vi "DB UI - Admin User.vi"() -> ()   [LabVIEW 2013]
uses:
  Controls/Combo Box.ctl
  <vilib>/Utility/miscctls.llb/LVRowAndColumnUnsignedTypeDef.ctl
  <vilib>/Utility/miscctls.llb/LVRowAndColumnTypeDef.ctl
  <vilib>/Utility/miscctls.llb/LVPointTypeDef.ctl
  Controls/DB - Admin User Query ColNames.ctl
  Controls/Logon - Enum.ctl
  Controls/Global SRTRS.vi
  Controls/Global CMS.vi
  Controls/Global AMS.vi
  <vilib>/addons/database/Connection.llb/DB Tools Open Connec (String).vi
  <vilib>/addons/database/Connection.llb/Conn Execute.vi
  <vilib>/addons/database/Recordset.llb/Rec Destroy - Connection.vi
  <vilib>/addons/database/Recordset.llb/Rec Fetch Recordset Data (R).vi
  <vilib>/addons/database/_DB Variant To Data/Database Variant To Data.xnode
  <vilib>/addons/database/NI_Database_API.lvlib
panel:
  in  "Application":string
  in  "List [CaptionOnly]":string caption="List"
  in  "Tab Control":enum32{"Debug"}(tab)
  in  "DB.Config.UserGroup":string="SRTRS.Config.UserGroup"
  in  "DB.Config.UserGroupRelation":string="SRTRS.Config.UserGroupRelation"
  out "Password Matched":bool
  out "Password Count Valid":bool
  out "Email Valid":bool
  out "MHandler":errorcluster
  out "Connection Information":T1={"Connection "="SQL Server 32bit HPEnvy", "Username"="admin", "Password"="admin123"}
  in  "Stop Button":bool
  out "Statemachine":errorcluster
  in  "# of Columns":i32=9
  out "Primary Keys":string[](array[string])=["OrderNo"]
  out "Foreign Keys":string[](array[string])=["OrderNo"]
  in  "Next Button":bool
  in  "Previous Button":bool
  out "1st Primary KEY":string
  in  "Last Button":bool
  in  "First Button":bool
  out "datetime string":string
  out "Changed":bool
  out "SQL Query":string
  in  "Include Inactive":bool=TRUE
  out "Extra Event From \"Select Foreign Key\"":bool
  out "IDENTITY COLUMN":string
  out "Close":errorcluster
  out "New Record in UI not in DB":bool
  out "Property Node":errorcluster
  out "DB":errorcluster
  in  "DB.Admin.Users":string="SRTRS.Admin.Users"
  out "Col INFO":string[][](array[string])
  in  "[PlantId]":string="4070"
  in  "DB.Config.TabUserAccess":string="SRTRS.Config.TabUserAccess" caption="DB.Schema.Table\nDB.Config.TabUserAccess"
  in  "DB.Config.UserStationAccess":string="SRTRS.Config.UserStationAccess"
  out "Col Hdrs[] DB Data Type":string[](array[string])
  in  "# of Rows":u32=11
  out "Col Hdrs[] DB Precision":string[](array[string])
  out "All Mandatory Fields Filled":bool
  in  "------------------------------------        User Details Header EVENTS     ------------------------------------":string caption="------------------------------------        Setup Tab     ------------------------------------"
  in  "------------------------------------------        Unused EVENTS     ----------------------------------------":string caption="------------------------------------        Setup Tab     ------------------------------------"
  out "Logon":errorcluster
  out "MCListBox":u32
  out "NewVal":i32
  out "User Details 2":u32
  out "Controls (Caption) that are blank (Unicode)":string[](array[string])
  in  "Save Enabled depends on \nFilled Mandatory Fields":bool
  in  "CellBG New Cells":u32(colorbox)=16777225
  in  "CellBG Unused Cells":u32(colorbox)=16777238
  in  "CellBG ColHdrs":u32(colorbox)=11776947
  in  "Ascending":bool
  out "transposed array":string[][](array[string])
  in  "DB.Config.Domain":string="SRTRS.Config.Domain"
  in  "DB.Config.Plant":string="SRTRS.Config.Plant"
  in  "Search User ID":T2
  in  "Save":bool caption="Setup Save"
  in  "New":bool caption="Setup Save"
  in  "User Details":T3 caption="Record"
  in  "Current Record":i32 caption="No."
  out "Record Count":i32
  in  "Multicolumn Listbox":i32(listbox)=3
  # "Cannot be placed in Tab, becasue calling VI only looking for non-Tabs."
  # "/"
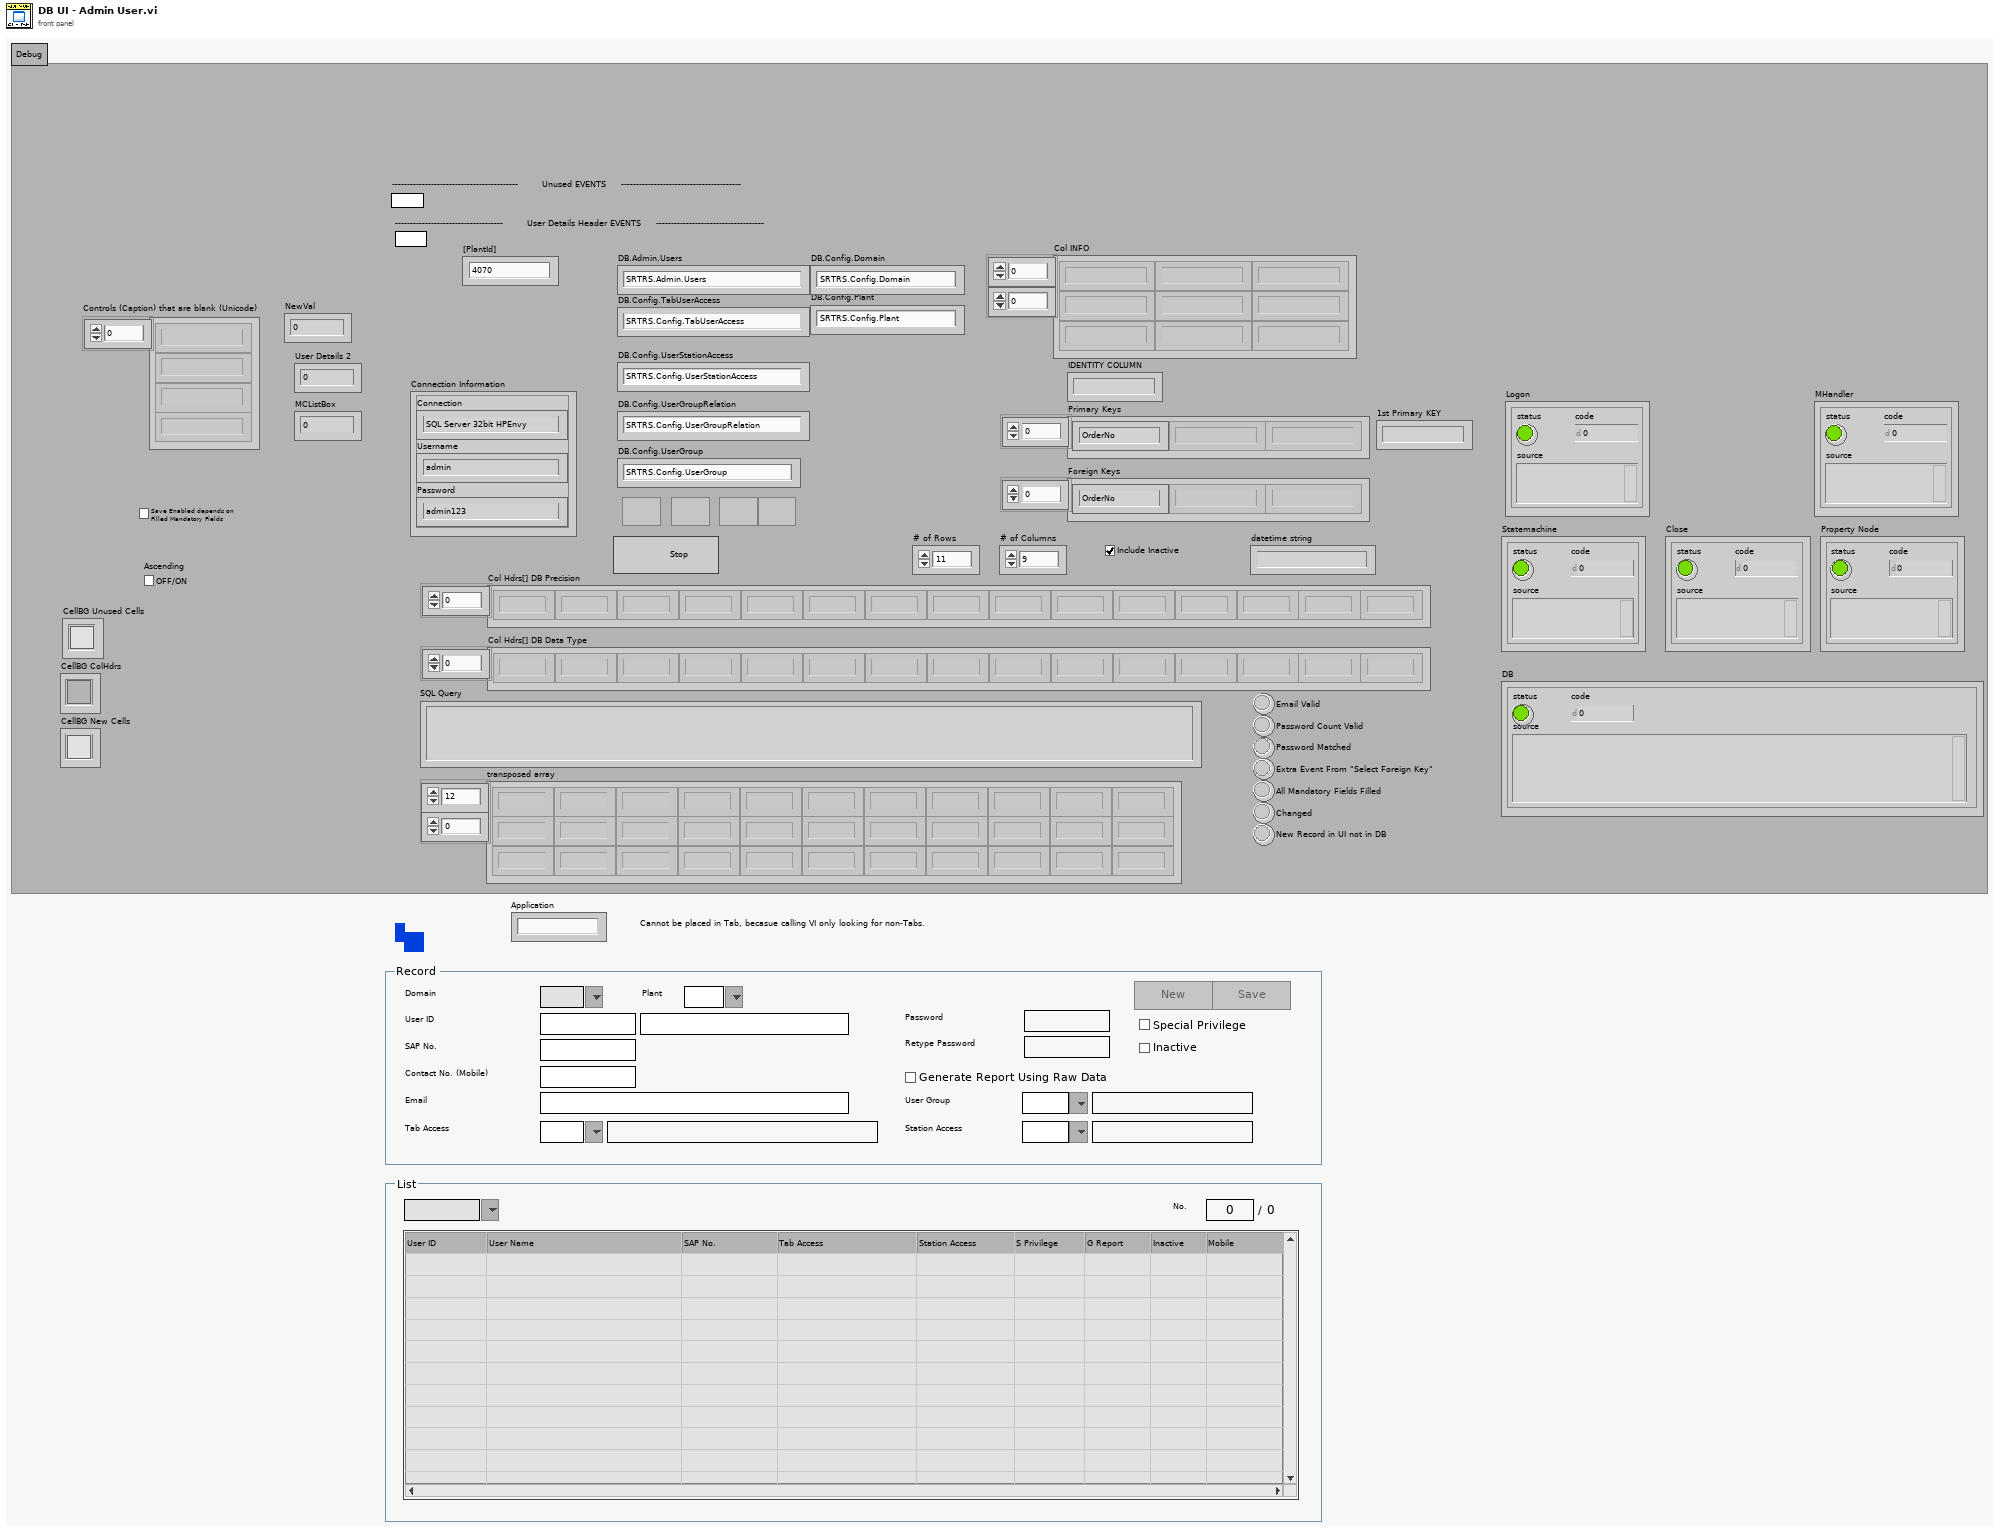
[diagram p1: front panel]
types:
  T1 = cluster{"Connection ":string, "Username":string, "Password":string}
  T2 = typedef "Combo Box.ctl" = string
  T3 = cluster{"Domain ID":T2, "User ID":string, "User Name":string, "SAP No.":string, "Plant ID":T2, "Mobile":string, "Email":string, "Tab Access ID":T2, "Tab Access":string, "Password":string, "Retype Password":string, "G Report":bool, "S Privilege":bool, "Inactive":bool, "Station Access ID":T2, "Station Access":string, "User Group ID":T2, "User Group":string}
  T4 = typedef "LVPointTypeDef.ctl" = cluster{"Horizontal":i16, "Vertical":i16}
  T5 = typedef "LVRowAndColumnUnsignedTypeDef.ctl" = cluster{"Row":u32, "Column":u32}
  T6 = enum8{"Enabled", "Disabled", "Disabled and Grayed Out"}
  T7 = typedef "DB - Admin User Query ColNames.ctl" = enum16{"PlantId", "UserId", "UserName", "DomainId", "SapNo", "MobileNo", "Email", "TabAccessId", "TabDescription", "StationAccessId", "StationDescription", "UserGroupId", "UserGroupDescription", "SpecialPrivilege", "RawDataReport", "Inactive"}
  T8 = typedef "LVRowAndColumnTypeDef.ctl" = cluster{"Row":i32, "Column":i32}
  T9 = typedef "Connection Information Cluster.ctl" = cluster{"Connection ":string, "Username":string, "Password":string}
  T10 = typedef "NI_Database_API.lvlib/Conn ObjectReference.ctl" = refnum<k1>
  T11 = typedef "Logon - Enum.ctl" = enum16{"PC username", "PC username INFO", "Hostname", "Check AD", "Logon", "QUIT"}
  T12 = typedef "DB - DB.Schema.Table.ctl" = cluster{"DB":string, "Schema":string, "Table":string}
  T13 = typedef "NI_Database_API.lvlib/Rec ObjectReference.ctl" = refnum<k1>
  T14 = typedef "eventvkey.ctl" = enum16{"ASCII", "Enter", "Return", "Shift", "Ctrl", "Alt", "Cmd", "Opt", "Caps", "NumLock", "Clear", "Break", "Up", "Down", "Left", "Right", "Insert", "Delete", "Home", "End", "PageUp", "PageDown", "Escape", "Help", "Pause", "ScrollLock", "F1", "F2", "F3", "F4", "F5", "F6", "F7", "F8", "F9", "F10", "F11", "F12", "F13", "F14", "F15", "F16", "F17", "F18", "F19", "F20", "F21", "F22", "F23", "F24", "Play", "VolumeUp", "VolumeDown", "Mute", "Two Byte Char"}
  T15 = cluster{"PC username":string, "Domain":string, "AD available":bool, "Username FOUND":bool, "Logon Full Name":string}
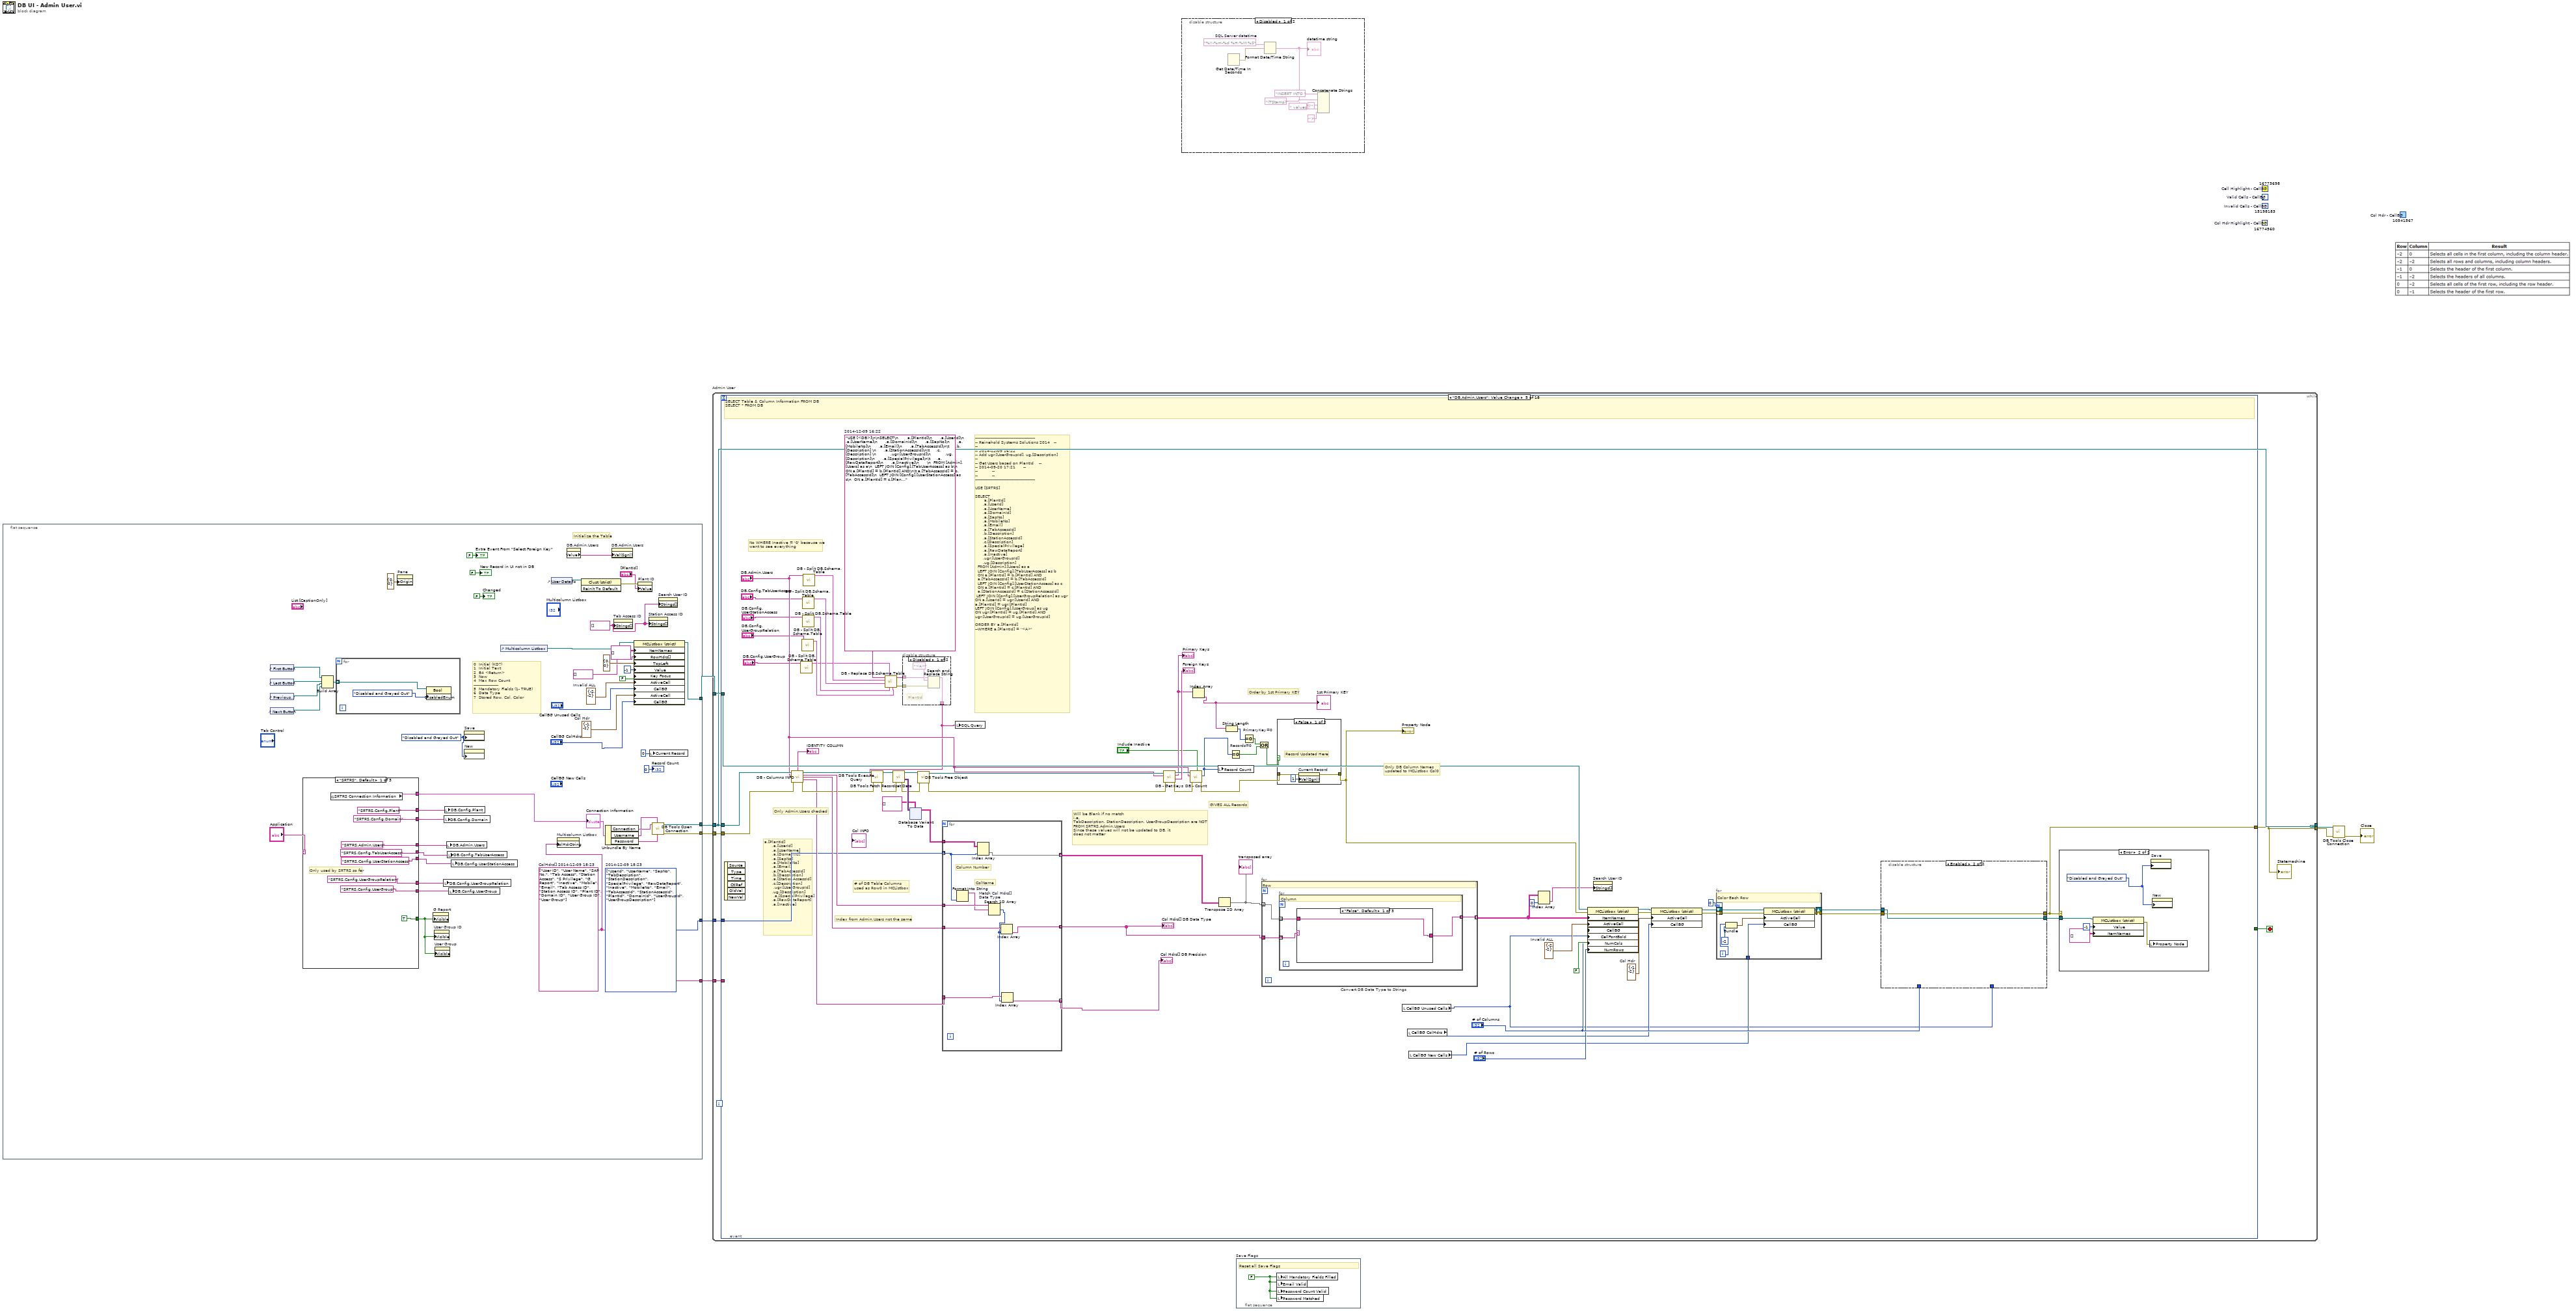
[diagram p0: block diagram]
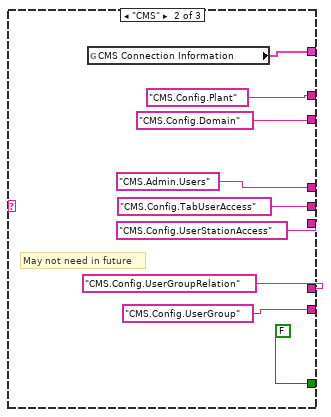
[diagram p3: hidden frame]
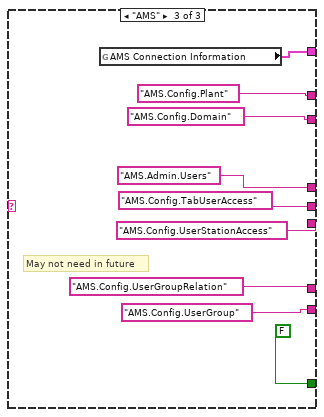
[diagram p4: hidden frame]
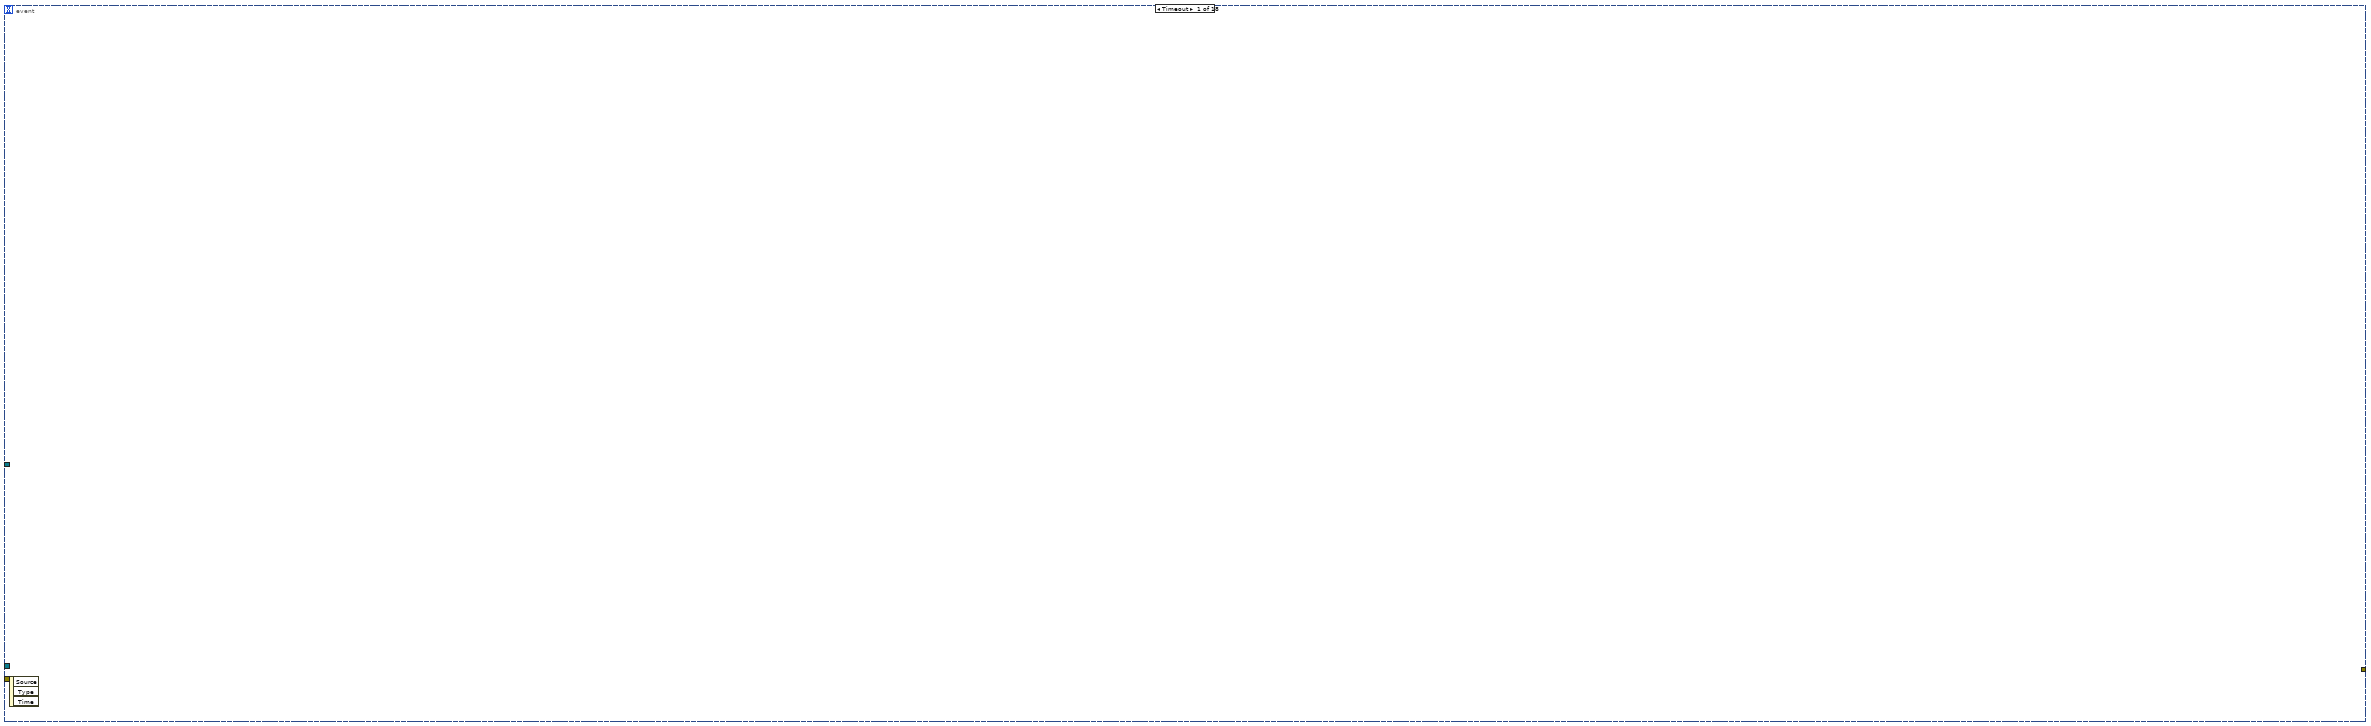
[diagram p5: hidden frame]
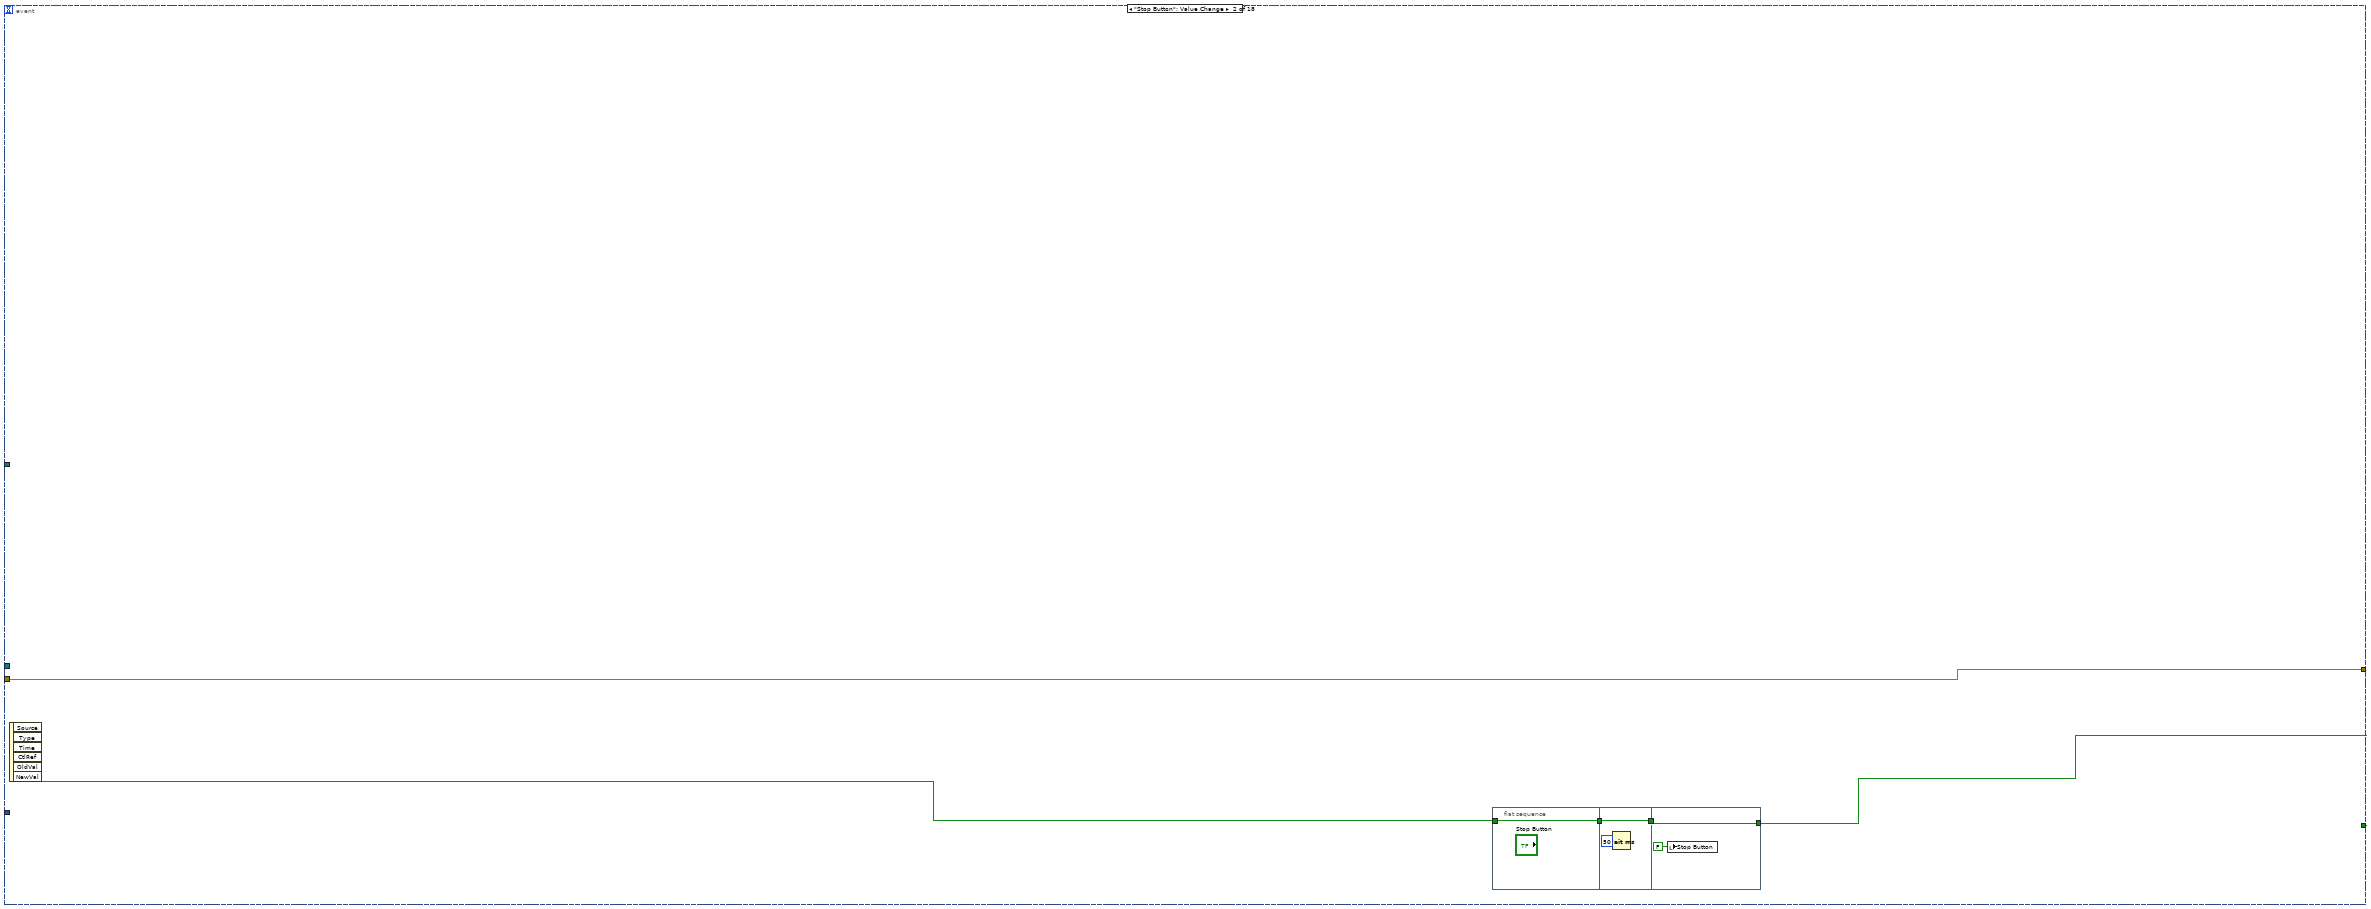
[diagram p6: hidden frame]
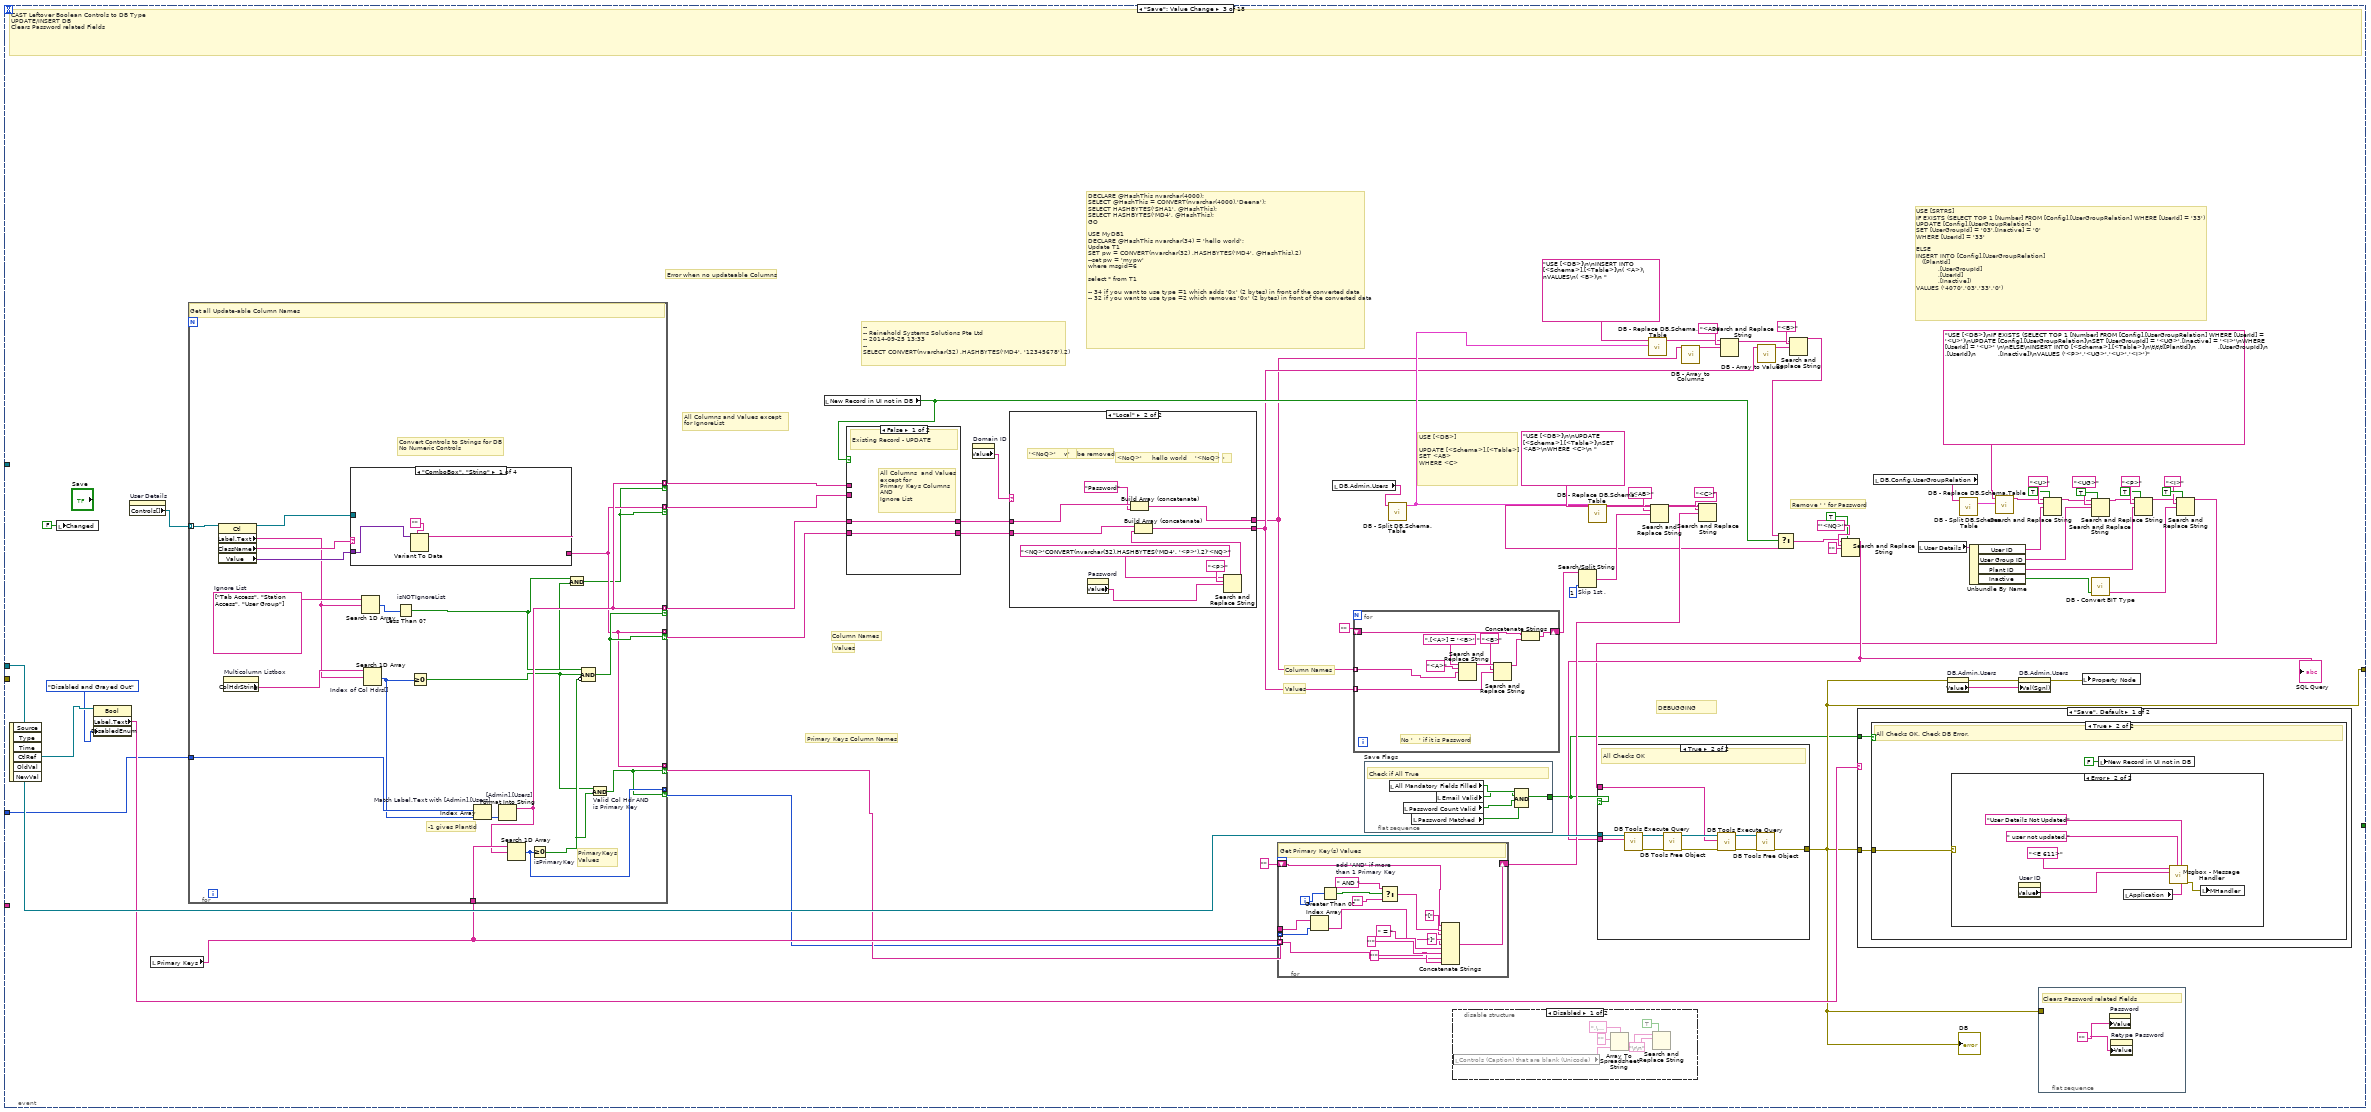
[diagram p7: hidden frame]
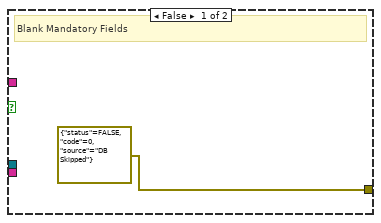
[diagram p9: hidden frame]
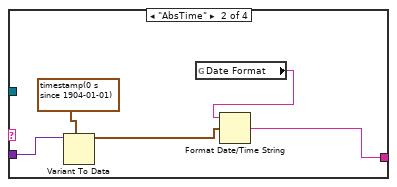
[diagram p11: hidden frame]
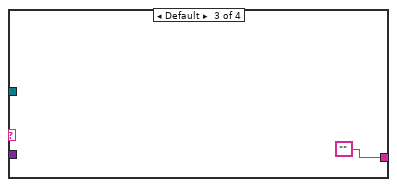
[diagram p12: hidden frame]
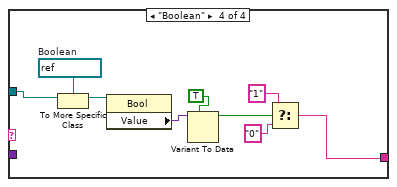
[diagram p13: hidden frame]
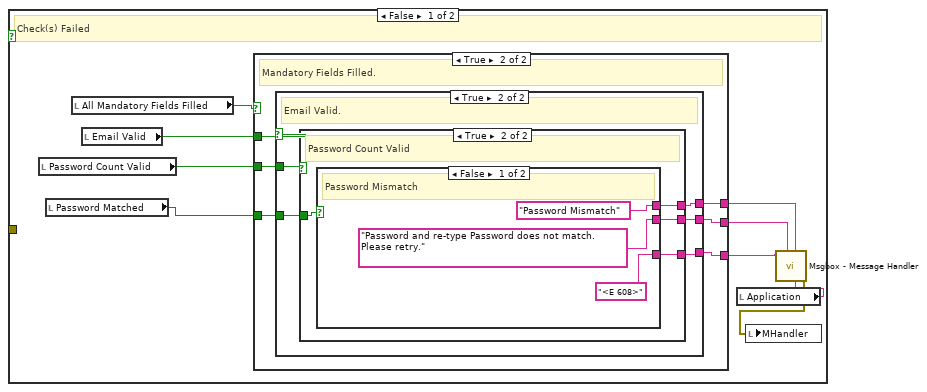
[diagram p15: hidden frame]
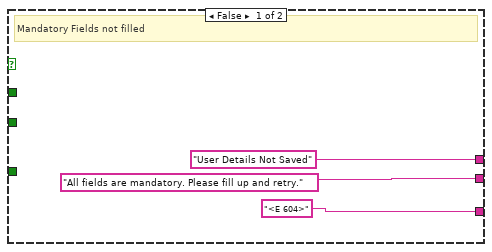
[diagram p16: hidden frame]
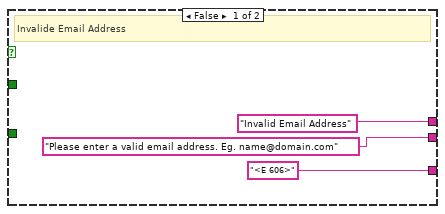
[diagram p17: hidden frame]
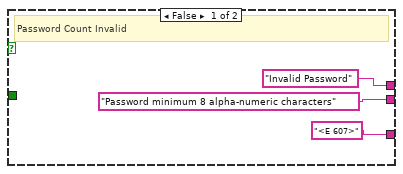
[diagram p18: hidden frame]
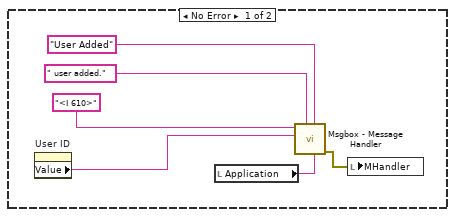
[diagram p20: hidden frame]
diagram:
  (unwired) u32 10541567  # Col Hdr - CellBG
  (unwired) u32 16777226  # Valid Cells - CellBG
  (unwired) u32 15198183  # Invalid Cells - CellBG
  (unwired) u32 16774560  # Col Hdr Highlight - CellBG
  (unwired) u32 16773698  # Cell Highlight - CellBG
  n1 = flat-sequence {
    tunnel: [w50] -> w8
    tunnel: [w29] -> w5
    tunnel: [w48] -> w4
    tunnel: [w12] -> w2
    tunnel: [w25] -> w1
    frame #0 {
      w12 = T7[] [enum."UserId", enum."UserName", enum."SapNo", enum."TabDescription", enum."StationDescription", enum."SpecialPrivilege", enum."RawDataReport", enum."Inactive", enum."MobileNo", enum."Email", enum."TabAccessId", enum."StationAccessId", enum."PlantId", enum."DomainId", enum."UserGroupId", enum."UserGroupDescription"] items=["PlantId", "UserId", "UserName", "DomainId", "SapNo", "MobileNo", "Email", "TabAccessId", "TabDescription", "StationAccessId", "StationDescription", "UserGroupId", "UserGroupDescription", "SpecialPrivilege", "RawDataReport", "Inactive"]  # 2014-12-09 18:23
      w24 = string[] [] ("Strings []")
      w25 = string[] ["User ID", "User Name", "SAP No.", "Tab Access", "Station Access", "S Privilege", "G Report", "Inactive", "Mobile", "Email", "Tab Access ID", "Station Access ID", "Plant ID", "Domain ID", "User Group ID", "User Group"]  # ColHdrs[] 2014-12-09 18:23
      w30 = T8 {"Row"=-1, "Column"=-2}  # Col Hdr
      w31 = T8 {"Row"=-2, "Column"=-2}  # Invalid ALL
      w38 = T6."Disabled and Grayed Out" ("Disabled")
      # "Initialize the Table"
      # "0  Initial (KD?)\n1  Initial Text\n2  B4 <Return>\n3  Now\n4  Max Row Count\n-------------------\n5  Mandatory Fields (1- TRUE)\n6  Data Type\n7  Stored Row, Col, Color"
      n2 = control-ref of="First Button"() -> (w44:refnum<vi>)
      n3 = control-ref of="Last Button"() -> (w43:refnum<vi>)
      n4 = control-ref of="Previous Button"() -> (w42:refnum<vi>)
      n5 = control-ref of="Next Button"() -> (w41:refnum<vi>)
      n6 = case shown="\"SRTRS\", Default" "Application" {
        tunnel: [w62 w71 w75] -> w20
        tunnel: ["SRTRS.Admin.Users" ("DB.Schema.Table\nDB.Admin.Users") "CMS.Admin.Users" ("DB.Schema.Table\nDB.Admin.Users") "AMS.Admin.Users" ("DB.Schema.Table\nDB.Admin.Users")] -> w19
        tunnel: ["SRTRS.Config.UserStationAccess" ("DB.Schema.Table\nDB.Config.UserStationAccess") "CMS.Config.UserStationAccess" ("DB.Schema.Table\nDB.Config.UserStationAccess") "AMS.Config.UserStationAccess" ("DB.Schema.Table\nDB.Config.UserStationAccess")] -> w16
        tunnel: ["SRTRS.Config.TabUserAccess" ("DB.Schema.Table\nDB.Config.TabUserAccess") "CMS.Config.TabUserAccess" ("DB.Schema.Table\nDB.Config.TabUserAccess") "AMS.Config.TabUserAccess" ("DB.Schema.Table\nDB.Config.TabUserAccess")] -> w15
        tunnel: [TRUE FALSE FALSE] -> w9
        tunnel: ["SRTRS.Config.UserGroupRelation" ("DB.Config.UserGroup") "CMS.Config.UserGroupRelation" ("DB.Config.UserGroup") "AMS.Config.UserGroupRelation" ("DB.Config.UserGroup")] -> w14
        tunnel: ["SRTRS.Config.UserGroup" ("DB.Config.UserGroup") "CMS.Config.UserGroup" ("DB.Config.UserGroup") "AMS.Config.UserGroup" ("DB.Config.UserGroup")] -> w13
        tunnel: ["SRTRS.Config.Plant" ("DB.Config.Plant") "CMS.Config.Plant" ("DB.Config.Plant") "AMS.Config.Plant" ("DB.Config.Plant")] -> w11
        tunnel: ["SRTRS.Config.Domain" ("DB.Config.Domain") "CMS.Config.Domain" ("DB.Config.Domain") "AMS.Config.Domain" ("DB.Config.Domain")] -> w10
        frame "SRTRS", Default {
          # "Only used by SRTRS so far"
          n7 = global read "Global SRTRS.vi" "SRTRS Connection Information"() -> (w62:T9)
        }
        frame "CMS" {
          # "May not need in future"
          n8 = global read "Global CMS.vi" "CMS Connection Information"() -> (w71:T9)
        }
        frame "AMS" {
          # "May not need in future"
          n9 = global read "Global AMS.vi" "AMS Connection Information"() -> (w75:T9)
        }
      }
      "Connection Information" <- w20
      n10 = Build Array(w44, w43, w42, w41) -> (w45:refnum<vi>[])
      n11 = for {
        tunnel: w45 -> [w82] mode=indexing
        n12 = property class="Bool"(reference=w82, "DisabledEnum"=T6."Disabled and Grayed Out" ("Disabled")) -> ()  [unwired: 1 in, 2 out]
      }
      n13 = property on="Pane" class="Pane"("Origin"=T4 {"Horizontal"=0, "Vertical"=0}) -> ()  [unwired: 2 in, 2 out]
      n14 = property on="G Report" class="Bool (strict)"("Visible"=w9) -> ()  [unwired: 2 in, 2 out]
      n15 = property on="User Group ID" class="CmbBox (strict)"("Visible"=w9) -> ()  [unwired: 2 in, 2 out]
      n16 = property on="User Group" class="Str"("Visible"=w9) -> ()  [unwired: 2 in, 2 out]
      n17 = local write "DB.Config.UserGroupRelation"(w14) -> ()
      n18 = local write "DB.Config.Domain"(w10) -> ()
      n19 = local write "DB.Config.Plant"(w11) -> ()
      n20 = local write "DB.Admin.Users"(w19) -> ()
      n21 = local write "DB.Config.TabUserAccess"(w15) -> ()
      n22 = local write "DB.Config.UserGroup"(w13) -> ()
      n23 = local write "DB.Config.UserStationAccess"(w16) -> ()
      n24 = property on="Save" class="Bool"("DisabledEnum"=w38) -> ()  [unwired: 2 in, 2 out]
      n25 = property on="New" class="Bool"("DisabledEnum"=w38) -> ()  [unwired: 2 in, 2 out]
      n26 = control-ref of="Multicolumn Listbox"() -> (w28:refnum<vi>)
      n27 = control-ref of="User Details"() -> (w27:refnum<vi>)
      n28 = property on="Multicolumn Listbox" class="MCListbox (strict)"("ColHdrString"=w25) -> ()  [unwired: 2 in, 2 out]
      n29 = property on="DB.Admin.Users" class="Str"() -> ("Value"=w37:string)  [unwired: 2 in, 2 out]
      n30 = invoke class="Clust (strict)" method="Reinit To Default"(reference=w27) -> (error out=w26:errorcluster)  [unwired: 2 in, 2 out]
      n31 = Unbundle By Name(w20) -> ("Connection"=w53:string, "Username"=w52:string, "Password"=w51:string)
      n32 = property on="DB.Admin.Users" class="Str"("Val(Sgnl)"=w37) -> ()  [unwired: 2 in, 2 out]
      n33 = property on="Tab Access ID" class="CmbBox (strict)"("Strings[]"=w24) -> ()  [unwired: 2 in, 2 out]
      n34 = property on="Property Node" class="MCListbox (strict)"(reference=w28, "ItemNames"=string[][] [] ("Item Names"), "RowHdrs[]"=string[] [] ("Item Names"), "TopLeft"=T5 {"Row"=0, "Column"=0} ("Top Left Visible Cell"), "Value"=-1, "Key Focus"=FALSE, "ActiveCell"=w31, "CellBG"="CellBG Unused Cells", "ActiveCell"=w30, "CellBG"="CellBG ColHdrs") -> (reference out=w29:refnum<vi>)  [unwired: 1 in, 1 out]
      n35 = property on="Plant ID" class="CmbBox (strict)"(error in=w26, "Value"="[PlantId]") -> ()  [unwired: 1 in, 2 out]
      n36 = property on="Station Access ID" class="CmbBox (strict)"("Strings[]"=w24) -> ()  [unwired: 2 in, 2 out]
      n37 = local write "Current Record"(0 ("Current Record")) -> ()
      n38 = call-poly <vilib>:"DB Tools Open Connection.vi"("password"=w51, "userID"=w52, "connection information"=w53) -> ("error out"=w48:errorcluster, "connection reference"=w50:T10)  [unwired: 5 in]
      n39 = property on="Search User ID" class="CmbBox (strict)"("Strings[]"=w24) -> ()  [unwired: 2 in, 2 out]
      "Extra Event From \"Select Foreign Key\"" <- FALSE ("Extra Event From \"Select Foreign Key Value Changed\"")
      "Record Count" <- 0 ("Record Count")
      "New Record in UI not in DB" <- FALSE ("New Record in UI not in DB")
      "Changed" <- FALSE ("Changed")
    }
  }
  n40 = while "Admin User" {
    tunnel: w8 -> [w86]
    tunnel: [w86] -> w7
    tunnel: [w85] -> w6
    tunnel: w4 -> [w88]
    tunnel: w5 -> [w87]
    tunnel: w2 -> [w84]
    tunnel: w1 -> [w83]
    stop <- w89 stop-if-true
    n41 = event shown="[4] \"DB.Admin.Users\": Value Change" {
      selector: _ -> [_ _ _ _ _ _ _ _ _ _ _ _ _ _ _ _ _ _]
      dyn-events: _ -> [_ _ _ _ _ _ _ _ _ _ _ _ _ _ _ _ _ _]
      timeout: _ -> [_ _ _ _ _ _ _ _ _ _ _ _ _ _ _ _ _ _]
      tunnel: [_ w92 _ _ _ _ _ _ _ _ _ _ _ _ _ _ _ _] -> w89
      tunnel: w86 -> [_ _ w173 _ w405 _ _ _ _ _ w676 w745 _ _ _ _ _ w1053]
      tunnel: [_ w94 w123 _ w392 _ w555 _ _ _ w654 _ _ _ _ _ _ _] -> w85
      tunnel: w88 -> [_ w94 _ _ w404 _ w556 _ _ _ _ _ _ _ _ _ _ w1052]
      tunnel: w87 -> [_ _ _ _ w413 w537 w554 _ _ _ _ _ _ _ w875 w929 _ _]
      tunnel: w84 -> [_ _ w144 _ w350 _ _ _ _ _ w665 w766 _ _ _ _ _ _]
      tunnel: w83 -> [_ _ _ _ _ _ _ _ _ _ w668 w769 _ _ _ _ _ _]
      event Timeout {
        n42 = event-data() -> ()  [unwired: 1 in, 3 out]
      }
      event "Stop Button": Value Change {
        n43 = event-data() -> ("NewVal"=w93:bool)  [unwired: 1 in, 5 out]
        n44 = flat-sequence {
          tunnel: w93 -> [w95]
          tunnel: [w95] -> w90
          tunnel: [w96] -> w91
          tunnel: w90 -> [w96]
          tunnel: [w98] -> w92
          tunnel: w91 -> [w98]
          frame #0 {
          }
          frame #1 {
            n45 = Wait (ms)(milliseconds to wait=u32 50) -> ()  [unwired: 1 out]
          }
          frame #2 {
            n46 = local write "Stop Button"(FALSE ("Stop Button")) -> ()
          }
        }
      }
      event "Save": Value Change {
        # "DEBUGGING"
        # "USE [SRTRS]\nIF EXISTS (SELECT TOP 1 [Number] FROM [Config].[UserGroupRelation] WHERE [UserId] = '33')\nUPDATE [Config].[UserGroupRelation]\nSET [UserGroupId] = '03',[Inactive] = '0'\nWHERE [UserId] = '33' \n\nELSE\nINSERT INTO [Config].[UserGroupRelation]\n\t\t\t([PlantId]\n           ,[UserGroupId]\n           ,[UserId]\n           ,[Inactive])\nVALUES ('4070','03','33','0')"
        # "--\n-- Reinehold Systems Solutions Pte Ltd\n-- 2014-09-25 13:33\n--\nSELECT CONVERT(nvarchar(32) ,HASHBYTES('MD4', '12345678'),2)"
        # "All Columns and Values except\nfor IgnoreList"
        # "Primary Keys Column Names"
        # "Values"
        # "Column Names"
        # "Remove ' ' for Password"
        # "DECLARE @HashThis nvarchar(4000);\nSELECT @HashThis = CONVERT(nvarchar(4000),'Deena');\nSELECT HASHBYTES('SHA1', @HashThis);\nSELECT HASHBYTES('MD4', @HashThis);\nGO\n\nUSE MyDB1\nDECLARE @HashThis nvarchar(34) = 'hello world';\nUpdate T1\nSET pw = CONVERT(nvarchar(32) ,HASHBYTES('MD4', @HashThis),2)\n--set pw = 'mypw'\nwhere msgid=6\n\nselect * from T1\n\n-- 34 if you want to use type =1 which adds '0x' (2 bytes) in front of the converted data\n-- 32 if you want to use type =2 which removes '0x' (2 bytes) in front of the converted data"
        # "Values"
        # "Column Names"
        # "Error when no updateable Columns"
        # "USE [<DB>]\n\nUPDATE [<Schema>].[<Table>]\nSET <AB>\nWHERE <C>"
        # "CAST Leftover Boolean Controls to DB Type\nUPDATE/INSERT DB\nClears Password related Fields"
        n47 = event-data() -> ("CtlRef"=w160:refnum<vi>)  [unwired: 1 in, 5 out]
        n48 = local write "Changed"(FALSE ("Changed")) -> ()
        n49 = property class="Bool"(reference=w160, "DisabledEnum"=T6."Disabled and Grayed Out" ("Disabled")) -> ("Label.Text"=w146:string)  [unwired: 1 in, 2 out]
        n50 = property on="User Details" class="Clust (strict)"() -> ("Controls[]"=w138:refnum<vi>[])  [unwired: 2 in, 2 out]
        n51 = local read "Primary Keys"() -> (w161:string[])
        n52 = for {
          tunnel: [w214] -> w137 mode=indexing if=w223
          tunnel: w161 -> [w222]
          tunnel: w138 -> [w228] mode=indexing
          tunnel: w144 -> [w226]
          tunnel: [w213] -> w136 mode=indexing if=w223
          tunnel: [w213] -> w143 mode=indexing if=w215
          tunnel: [w216] -> w142 mode=indexing if=w215
          tunnel: [w214] -> w140 mode=indexing if=w211
          tunnel: [w213] -> w139 mode=indexing if=w211
          w220 = string[] ["Tab Access", "Station Access", "User Group"]  # Ignore List
          # "Convert Controls to Strings for DB\nNo Numeric Controls"
          # "PrimaryKeys\nValues"
          # "-1 gives PlantId"
          # "Get all Update-able Column Names"
          n53 = property class="Ctl"(reference=w228) -> (reference out=w208:refnum<vi>, "Label.Text"=w219:string, "ClassName"=w225:string, "Value"=w224:variant)  [unwired: 1 in, 1 out]
          n54 = property on="Multicolumn Listbox" class="MCListbox (strict)"() -> ("ColHdrString"=w227:string[])  [unwired: 2 in, 2 out]
          n55 = case shown="\"ComboBox\", \"String\"" w225 {
            tunnel: w224 -> [w229 w232 _ _]
            tunnel: [w230 w233 "" w238] -> w213
            tunnel: w208 -> [_ _ _ w246]
            frame "ComboBox", "String" {
              n56 = Variant To Data(type="", Variant=w229) -> (data=w230:string)  [unwired: 1 in, 1 out]
            }
            frame "AbsTime" {
              n57 = Variant To Data(type=timestamp(0 s since 1904-01-01), Variant=w232) -> (data=w235:timestamp)  [unwired: 1 in, 1 out]
              n58 = global read "Global SRTRS.vi" "Date Format"() -> (w234:string)
              n59 = Format Date/Time String(time format string (%c)=w234, seconds (now)=w235) -> (date/time string=w233:string)  [unwired: 1 in]
            }
            frame Default {
            }
            frame "Boolean" {
              w245 = refnum<vi> refnum  # Boolean
              n60 = To More Specific Class(target class=w245, reference=w246) -> (specific class reference=w244:refnum<vi>)  [unwired: 1 in, 1 out]
              n61 = property class="Bool"(reference=w244) -> ("Value"=w239:variant)  [unwired: 1 in, 2 out]
              n62 = Variant To Data(type=TRUE, Variant=w239) -> (data=w242:bool)  [unwired: 1 in, 1 out]
              n63 = Select(t="1", s=w242, f="0") -> (s? t:f=w238:string)
            }
          }
          n64 = Search 1D Array(1D array=w220, element=w219) -> (index of element=w221:i32)  [unwired: 1 in]
          n65 = Search 1D Array "Index of Col Hdrs[]"(1D array=w227, element=w219) -> (index of element=w209:i32)  [unwired: 1 in]
          n66 = Less Than 0? "isNOTIgnoreList"(x=w221) -> (x < 0?=w212:bool)
          n67 = Greater Or Equal To 0?(x=w209) -> (x >= 0?=w210:bool)
          n68 = Index Array "Match Label.Text with [Admin].[Users]"(array=w226, index=w209) -> (element=w218:T7)
          n69 = Format Into String "[Admin].[Users]"(w218) -> (resulting string=w214:string)  [unwired: 3 in, 1 out]
          n70 = Search 1D Array(1D array=w222, element=w214) -> (index of element=w216:i32)  [unwired: 1 in]
          n71 = Greater Or Equal To 0? "isPrimaryKey"(x=w216) -> (x >= 0?=w217:bool)
          n72 = Compound Arithmetic op=AND(w212, w210) -> (w211:bool)
          n73 = Compound Arithmetic op=AND(w212, w210, invert w217) -> (w223:bool)
          n74 = Compound Arithmetic op=AND "Valid Col Hdr AND\nis Primary Key"(w210, w217) -> (w215:bool)
        }
        n75 = local read "New Record in UI not in DB"() -> (w141:bool)
        n76 = case shown="False" w141 {
          tunnel: w140 -> [_ w250]
          tunnel: w139 -> [_ w249]
          tunnel: w137 -> [w248 _]
          tunnel: w136 -> [w247 _]
          tunnel: [w248 w250] -> w134
          tunnel: [w247 w249] -> w133
          frame False {
            # "All Columns  and Values\nexcept for\nPrimary Keys Columns\nAND\nIgnore List"
            # "Existing Record - UPDATE"
          }
          frame True {
            # "All Columns and Values\nIncluding Primary Keys\nExcluding Ignore List"
            # "New Record - INSERT"
          }
        }
        n77 = property on="Domain ID" class="CmbBox (strict)"() -> ("Value"=w135:T2)  [unwired: 2 in, 2 out]
        n78 = case shown="\"Local\"" w135 {
          tunnel: w134 -> [w198 w207]
          tunnel: [w198 w206] -> w124
          tunnel: w133 -> [w197 w204]
          tunnel: [w197 w203] -> w132
          frame "False", Default {
          }
          frame "Local" {
            # "'<NoQ>'    will be removed"
            # "'"
            # "'"
            # "<NoQ>'     hello world    '<NoQ>"
            n79 = property on="Password" class="Str"() -> ("Value"=w201:string)  [unwired: 2 in, 2 out]
            n80 = Build Array (concatenate)(w207, "Password") -> (w206:string[])
            n81 = Search and Replace String(input string="<NQ>'CONVERT(nvarchar(32),HASHBYTES('MD4', '<P>'),2)'<NQ>", search string="<P>", replace string=w201) -> (result string=w200:string)  [unwired: 5 in, 3 out]
            n82 = Build Array (concatenate)(w204, w200) -> (w203:string[])
          }
        }
        n83 = for {
          tunnel: w161 -> [w311]
          shift-right: [w318] -> w162
          shift-left: "" -> [w313]
          tunnel: w143 -> [w312] mode=indexing
          tunnel: w142 -> [w310] mode=indexing
          i -> [w319]
          w316 = " AND "  # add 'AND' if more  than 1 Primary Key
          # "Get Primary Key(s) Values"
          n84 = Index Array(array=w311, index=w310) -> (element=w309:string)
          n85 = Greater Than 0?(x=w319) -> (x > 0?=w317:bool)
          n86 = Select(t=w316, s=w317, f="") -> (s? t:f=w314:string)
          n87 = Concatenate Strings(w313, w314, "[" ("string"), w309, "]" ("string"), " = " ("string"), "'" ("string"), w312, "'" ("string")) -> (w318:string)
        }
        n88 = local read "DB.Admin.Users"() -> (w145:string)
        n89 = for {
          tunnel: w132 -> [w328] mode=indexing
          shift-right: [w325] -> w170
          shift-left: "" -> [w327]
          tunnel: w124 -> [w324] mode=indexing
          # "No '   ' if it is Password"
          n90 = Search and Replace String(input string=",[<A>] = '<B>' ", search string="<A>", replace string=w324) -> (result string=w329:string)  [unwired: 5 in, 3 out]
          n91 = Search and Replace String(input string=w329, search string="<B>", replace string=w328) -> (result string=w326:string)  [unwired: 5 in, 3 out]
          n92 = Concatenate Strings(w327, w326) -> (w325:string)
        }
        n93 = flat-sequence "Save Flags" {
          tunnel: [w178] -> w100
          frame #0 {
            # "Check if All True"
            n94 = local read "All Mandatory Fields Filled"() -> (w177:bool)
            n95 = local read "Password Count Valid"() -> (w175:bool)
            n96 = local read "Password Matched"() -> (w174:bool)
            n97 = local read "Email Valid"() -> (w176:bool)
            n98 = Compound Arithmetic op=AND(w177, w176, w175, w174) -> (w178:bool)
          }
        }
        n99 = call "DB - Split DB.Schema.Table.vi"("DB.Schema.Table"=w145) -> ("DB.Schema.Table"=w148:T12)  [unwired: 10 in]
        n100 = disable-structure shown="Disabled" {
          frame Disabled {
            n101 = local read "Controls (Caption) that are blank (Unicode)"() -> (w179:string[])
            n102 = Array To Spreadsheet String(delimiter (Tab)=",\u0000", array=w179, 3:"" ("format string")) -> (spreadsheet string=w182:string)
            n103 = Search and Replace String(replace all?=TRUE ("replace all? (F)"), input string=w182, search string="\r\n") -> ()  [unwired: 5 in, 4 out]
          }
          frame Enabled {
          }
        }
        n104 = Search/Split String "Skip 1st ,"(string=w170, offset (0)=1) -> (match + rest of string=w165:string)  [unwired: 1 in, 2 out]
        n105 = call "DB - Replace DB.Schema.Table.vi"("DB.Schema.Table"=w148, "string in"="USE [<DB>]\n\nUPDATE [<Schema>].[<Table>]\nSET <AB>\nWHERE <C>\n ") -> ("string out"=w167:string)  [unwired: 8 in, 1 out]
        n106 = call "DB - Replace DB.Schema.Table.vi"("DB.Schema.Table"=w148, "string in"="USE [<DB>]\n\nINSERT INTO [<Schema>].[<Table>]\n( <A>)\nVALUES\n( <B>)\n ") -> ("string out"=w149:string)  [unwired: 8 in, 1 out]
        n107 = Search and Replace String(input string=w167, search string="<AB>", replace string=w165) -> (result string=w164:string)  [unwired: 5 in, 3 out]
        n108 = call "DB - Array to Columns.vi"("Array"=w124) -> ("[Columns]"=w155:string)  [unwired: 10 in]
        n109 = Search and Replace String(input string=w164, search string="<C>", replace string=w162) -> (result string=w151:string)  [unwired: 5 in, 3 out]
        n110 = Search and Replace String(input string=w149, search string="<A>", replace string=w155) -> (result string=w152:string)  [unwired: 5 in, 3 out]
        n111 = call "DB - Array to Values.vi"("Array (0xFFFE autodetect)"=w132) -> ("<Values>"=w154:string)  [unwired: 10 in]
        n112 = Search and Replace String(input string=w152, search string="<B>", replace string=w154) -> (result string=w128:string)  [unwired: 5 in, 3 out]
        n113 = Select(t=w128, s=w141, f=w151) -> (s? t:f=w127:string)
        n114 = Search and Replace String(replace all?=TRUE ("replace all? (F)"), input string=w127, search string="'<NQ>'", replace string="" ("replace string (\"\")")) -> (result string=w126:string)  [unwired: 4 in, 3 out]
        "SQL Query" <- w126
        n115 = local read "DB.Config.UserGroupRelation"() -> (w121:string)
        n116 = local read "User Details"() -> (w110:T3)
        n117 = call "DB - Split DB.Schema.Table.vi"("DB.Schema.Table"=w121) -> ("DB.Schema.Table"=w120:T12)  [unwired: 10 in]
        n118 = Unbundle By Name(w110) -> ("User ID"=w109:string, "User Group ID"=w108:T2, "Plant ID"=w107:T2, "Inactive"=w102:bool)
        n119 = call "DB - Replace DB.Schema.Table.vi"("DB.Schema.Table"=w120, "string in"="USE [<DB>]\nIF EXISTS (SELECT TOP 1 [Number] FROM [Config].[UserGroupRelation] WHERE [UserId] = '<U>')\nUPDATE [Config].[UserGroupRelation]\nSET [UserGroupId] = '<UG>',[Inactive] = '<I>'\nWHERE [UserId] = '<U>' \n\nELSE\nINSERT INTO [<Schema>].[<Table>]\n\t\t\t([PlantId]\n           ,[UserGroupId]\n           ,[UserId]\n           ,[Inactive])\nVALUES ('<P>','<UG>','<U>','<I>')") -> ("string out"=w118:string)  [unwired: 8 in, 1 out]
        n120 = flat-sequence {
          tunnel: w123 -> [_]
          frame #0 {
            w185 = ""
            # "Clears Password related Fields"
            n121 = property on="Password" class="Str"("Value"=w185) -> ()  [unwired: 2 in, 2 out]
            n122 = property on="Retype Password" class="Str"("Value"=w185) -> ()  [unwired: 2 in, 2 out]
          }
        }
        n123 = Search and Replace String(replace all?=TRUE ("replace all? (F)"), input string=w118, search string="<U>", replace string=w109) -> (result string=w112:string)  [unwired: 4 in, 3 out]
        n124 = Search and Replace String(replace all?=TRUE ("replace all? (F)"), input string=w112, search string="<UG>", replace string=w108) -> (result string=w111:string)  [unwired: 4 in, 3 out]
        n125 = call "DB - Convert BIT Type.vi"("Boolean"=w102) -> ("BIT (eg Inactive)"=w101:string)  [unwired: 2 in, 2 out]
        n126 = Search and Replace String(replace all?=TRUE ("replace all? (F)"), input string=w111, search string="<P>", replace string=w107) -> (result string=w104:string)  [unwired: 4 in, 3 out]
        n127 = Search and Replace String(replace all?=TRUE ("replace all? (F)"), input string=w104, search string="<I>", replace string=w101) -> (result string=w103:string)  [unwired: 4 in, 3 out]
        n128 = case shown="True" w100 {
          tunnel: w173 -> [_ w196]
          tunnel: [errorcluster {"status"=FALSE, "code"=0, "source"="DB Skipped"} ("error out") w190] -> w123
          tunnel: w126 -> [_ w188]
          tunnel: w103 -> [_ w187]
          frame False {
            # "Blank Mandatory Fields"
          }
          frame True {
            # "All Checks OK"
            n129 = call-poly <vilib>:"DB Tools Execute Query.vi"("SQL query"=w188, "connection reference"=w196) -> ("error out"=w189:errorcluster, "recordset reference"=w195:T13)  [unwired: 6 in]
            n130 = call-poly <vilib>:"DB Tools Free Object.vi"("error in (no error)"=w189, "recordset reference"=w195) -> ("error out"=w192:errorcluster, "connection reference"=w191:T10)  [unwired: 8 in]
            n131 = call-poly <vilib>:"DB Tools Execute Query.vi"("error in (no error)"=w192, "SQL query"=w187, "connection reference"=w191) -> ("error out"=w194:errorcluster, "recordset reference"=w193:T13)  [unwired: 5 in]
            n132 = call-poly <vilib>:"DB Tools Free Object.vi"("error in (no error)"=w194, "recordset reference"=w193) -> ("error out"=w190:errorcluster)  [unwired: 8 in, 1 out]
          }
        }
        "DB" <- w123
        n133 = case shown="\"Save\", Default" w146 {
          tunnel: w123 -> [w252 _]
          tunnel: w100 -> [w251 _]
          frame "Save", Default {
            n134 = case shown="True" w251 {
              tunnel: w252 -> [_ w289]
              frame False {
                # "Check(s) Failed"
                n135 = local read "Password Count Valid"() -> (w256:bool)
                n136 = local read "Password Matched"() -> (w255:bool)
                n137 = local read "All Mandatory Fields Filled"() -> (w261:bool)
                n138 = local read "Email Valid"() -> (w260:bool)
                n139 = case shown="True" w261 {
                  tunnel: w260 -> [_ w270]
                  tunnel: ["User Details Not Saved" ("Short Description (When DB Not Available)") w269] -> w259
                  tunnel: ["All fields are mandatory. Please fill up and retry." ("Description (When DB Not Available)") w268] -> w258
                  tunnel: ["<E 604>" ("<.?....> Message Code") w267] -> w257
                  tunnel: w256 -> [_ w266]
                  tunnel: w255 -> [_ w265]
                  frame False {
                    # "Mandatory Fields not filled"
                  }
                  frame True {
                    # "Mandatory Fields Filled."
                    n140 = case shown="True" w270 {
                      tunnel: ["Invalid Email Address" ("Short Description (When DB Not Available)") w276] -> w269
                      tunnel: ["Please enter a valid email address. Eg. name@domain.com" ("Description (When DB Not Available)") w275] -> w268
                      tunnel: ["<E 606>" ("<.?....> Message Code") w274] -> w267
                      tunnel: w266 -> [_ w278]
                      tunnel: w265 -> [_ w277]
                      frame False {
                        # "Invalide Email Address"
                      }
                      frame True {
                        # "Email Valid."
                        n141 = case shown="True" w278 {
                          tunnel: w277 -> [_ w285]
                          tunnel: ["Invalid Password" w284] -> w276
                          tunnel: ["Password minimum 8 alpha-numeric characters" w282] -> w275
                          tunnel: ["<E 607>" w283] -> w274
                          frame False {
                            # "Password Count Invalid"
                          }
                          frame True {
                            # "Password Count Valid"
                            n142 = case shown="False" w285 {
                              tunnel: ["Password Mismatch" _] -> w284
                              tunnel: ["<E 608>" _] -> w283
                              tunnel: ["Password and re-type Password does not match. Please retry." _] -> w282
                              frame False {
                                # "Password Mismatch"
                              }
                              frame True {
                                # "Will not get here :)"
                                # "Password Match"
                              }
                            }
                          }
                        }
                      }
                    }
                  }
                }
                n143 = local read "Application"() -> (w254:string)
                n144 = call "Msgbox - Message Handler.vi"("Application (Default SRTRS)"=w254, "Short Description (When DB Not Available)"=w259, "Description (When DB Not Available)"=w258, "<.?....> Message Code"=w257) -> ("MHandler Error"=w253:errorcluster)  [unwired: 5 in, 2 out]
                n145 = local write "MHandler"(w253) -> ()
              }
              frame True {
                # "All Checks OK. Check DB Error."
                n146 = case shown="Error" w289 {
                  frame No Error {
                    n147 = property on="User ID" class="Str"() -> ("Value"=w294:string)  [unwired: 2 in, 2 out]
                    n148 = local read "Application"() -> (w291:string)
                    n149 = call "Msgbox - Message Handler.vi"("Application (Default SRTRS)"=w291, "Short Description (When DB Not Available)"="User Added" ("Description (When DB Not Available)"), "Description (When DB Not Available)"=" user added.", "Pre-Description"=w294, "<.?....> Message Code"="<I 610>" ("Description (When DB Not Available)")) -> ("MHandler Error"=w292:errorcluster)  [unwired: 4 in, 2 out]
                    n150 = local write "MHandler"(w292) -> ()
                  }
                  frame Error {
                    n151 = property on="User ID" class="Str"() -> ("Value"=w300:string)  [unwired: 2 in, 2 out]
                    n152 = local read "Application"() -> (w297:string)
                    n153 = call "Msgbox - Message Handler.vi"("Application (Default SRTRS)"=w297, "Short Description (When DB Not Available)"="User Details Not Updated" ("Description (When DB Not Available)"), "Description (When DB Not Available)"=" user not updated.", "Pre-Description"=w300, "<.?....> Message Code"="<E 611>" ("Description (When DB Not Available)")) -> ("MHandler Error"=w298:errorcluster)  [unwired: 4 in, 2 out]
                    n154 = local write "MHandler"(w298) -> ()
                  }
                }
                n155 = local write "New Record in UI not in DB"(FALSE ("New Record in UI not in DB")) -> ()
              }
            }
          }
          frame "Delete" {
            n156 = local read "Include Inactive"() -> (w303:bool)
            n157 = case shown="False" w303 {
              frame False {
                # "- 1 record"
                n158 = local read "Record Count"() -> (w306:i32)
                n159 = Decrement(x=w306) -> (x-1=w305:i32)
                n160 = local write "Record Count"(w305) -> ()
                n161 = Equal To 0?(x=w305) -> (x = 0?=w304:bool)
                n162 = case shown="True" w304 {
                  frame False {
                  }
                  frame True {
                    # "Refresh Table since NO record left"
                  }
                }
              }
              frame True {
                # "No Change"
              }
            }
          }
        }
        n163 = property on="DB.Admin.Users" class="Str"(error in=w123) -> (error out=w158:errorcluster, "Value"=w157:string)  [unwired: 1 in, 1 out]
        n164 = property on="DB.Admin.Users" class="Str"(error in=w158, "Val(Sgnl)"=w157) -> (error out=w147:errorcluster)  [unwired: 1 in, 1 out]
        n165 = local write "Property Node"(w147) -> ()
      }
      event "New": Value Change {
        n166 = event-data() -> ()  [unwired: 1 in, 6 out]
        n167 = local read "Application"() -> (w332:string)
        n168 = call "Msgbox - Message Handler.vi"("Application (Default SRTRS)"=w332, "Short Description (When DB Not Available)"="Create New User", "Description (When DB Not Available)"="All unsaved data will be lost. Do you want to proceed?", "<.?....> Message Code"="<W 601>") -> ("MHandler Error"=→"MHandler":errorcluster, "OK Out"=w334:bool)  [unwired: 5 in, 1 out]
        n169 = case shown="True" w334 {
          frame False {
          }
          frame True {
            n170 = control-ref of="User Details"() -> (w342:refnum<vi>)
            n171 = flat-sequence "Save Flags" {
              frame #0 {
                w344 = FALSE
                # "Reset all Save Flags"
                n172 = local write "All Mandatory Fields Filled"(w344) -> ()
                n173 = local write "Email Valid"(w344) -> ()
                n174 = local write "Password Count Valid"(w344) -> ()
                n175 = local write "Password Matched"(w344) -> ()
              }
            }
            n176 = invoke class="Clust (strict)" method="Reinit To Default"(reference=w342) -> (error out=w340:errorcluster)  [unwired: 2 in, 2 out]
            n177 = local read "New Record in UI not in DB"() -> (w341:bool)
            n178 = local write "All Mandatory Fields Filled"(FALSE ("All Mandatory Fields Filled")) -> ()
            n179 = property on="Plant ID" class="CmbBox (strict)"(error in=w340, "Value"="") -> ()  [unwired: 1 in, 2 out]
            n180 = case shown="False" w341 {
              frame False {
                n181 = local read "Record Count"() -> (w347:i32)
                n182 = local write "New Record in UI not in DB"(TRUE ("New Record in UI not in DB")) -> ()
                n183 = Increment(x=w347) -> (x+1=w346:i32)
                n184 = property on="Current Record" class="DigNum (strict)"("Value"=w346) -> ()  [unwired: 2 in, 2 out]
                n185 = local write "Record Count"(w346) -> ()
              }
              frame True {
                # "Already NEW so no need to add records"
              }
            }
            n186 = property on="Multicolumn Listbox" class="MCListbox (strict)"("Value"=-1 ("Multicolumn Listbox")) -> ()  [unwired: 2 in, 2 out]
          }
        }
      }
      event "DB.Admin.Users": Value Change {
        w379 = "USE [<DB>]\n\nSELECT\n       a.[PlantId]\n      ,a.[UserId]\n      ,a.[UserName]\n      ,a.[DomainId]\n      ,a.[SapNo]\n      ,a.[MobileNo]\n      ,a.[Email]\n      ,a.[TabAccessId]\n\t     ,b.[Description] \n      ,a.[StationAccessId]\n\t     ,c.[Description] \n           ,ugr.[UserGroupId]\n           ,ug.[Description]\n      ,a.[SpecialPrivilege]\n\t     ,a.[RawDataReport]\n      ,a.[Inactive]\n      \n  FROM [Admin].[Users] as a\n  LEFT JOIN [Config].[TabUserAccess] as b\n  ON a.[PlantId] = b.[PlantId] AND\n\t a.[TabAccessId] = b.[TabAccessId]\n  LEFT JOIN [Config].[UserStationAccess] as c\n  ON a.[PlantId] = c.[PlantId] AND\n\t a.[StationAccessId] = c.[StationAccessId]\n LEFT JOIN [Config].[UserGroupRelation] as ugr\nON a.[UserId] = ugr.[UserId] AND \na.[PlantId] = ugr.[PlantId]\nLEFT JOIN [Config].[UserGroup] as ug\nON ugr.[PlantId] = ug.[PlantId] AND\nugr.[UserGroupId] = ug.[UserGroupId]\n\nORDER BY a.[PlantId]\n--WHERE a.[PlantId] = '<A>'\n"  # 2014-12-09 16:22
        w406 = T8 {"Row"=-1, "Column"=-2}  # Col Hdr
        w417 = T8 {"Row"=-2, "Column"=-2}  # Invalid ALL
        # "a.[PlantId]\n      ,a.[UserId]\n      ,a.[UserName]\n      ,a.[DomainId]\n      ,a.[SapNo]\n      ,a.[MobileNo]\n      ,a.[Email]\n      ,a.[TabAccessId]\n\t     ,b.[Description] \n      ,a.[StationAccessId]\n\t     ,c.[Description] \n       ,ugr.[UserGroupId]\n      ,ug.[Description]      \n       ,a.[SpecialPrivilege]\n\t     ,a.[RawDataReport]\n      ,a.[Inactive]"
        # "Index from Admin.Users not the same"
        # "No WHERE Inactive = '0' because we\nwant to see everything"
        # "GIVES ALL Records"
        # "Will be Blank if no match\ni.e.\nTabDescription, StationDescription, UserGroupDescription are NOT \nFROM SRTRS.Admin.Users\nSince these values will not be updated to DB, it \ndoes not matter"
        # "----------------------------------------------\n-- Reinehold Systems Solutions 2014\t\t\t--\n--\n-- 2014-12-09 16:22\n-- Add ugr.[UserGroupId], ug.[Description]\n--\n-- Get Users based on PlantId\t\t\t\t--\n-- 2014-09-20 17:21\t\t\t\t\t\t--\n--\t\t\t\t\t\t\t\t\t\t\t--\n--\t\t\t\t\t\t\t\t\t\t\t--\n----------------------------------------------\n\nUSE [SRTRS]\n\nSELECT\n       a.[PlantId]\n      ,a.[UserId]\n      ,a.[UserName]\n      ,a.[DomainId]\n      ,a.[SapNo]\n      ,a.[MobileNo]\n      ,a.[Email]\n      ,a.[TabAccessId]\n\t     ,b.[Description] \n      ,a.[StationAccessId]\n\t     ,c.[Description] \n      ,a.[SpecialPrivilege]\n\t     ,a.[RawDataReport]\n      ,a.[Inactive]\n      ,ugr.[UserGroupId]\n      ,ug.[Description]\n  FROM [Admin].[Users] as a\n  LEFT JOIN [Config].[TabUserAccess] as b\n  ON a.[PlantId] = b.[PlantId] AND\n\t a.[TabAccessId] = b.[TabAccessId]\n  LEFT JOIN [Config].[UserStationAccess] as c\n  ON a.[PlantId] = c.[PlantId] AND\n\t a.[StationAccessId] = c.[StationAccessId]\n LEFT JOIN [Config].[UserGroupRelation] as ugr\nON a.[UserId] = ugr.[UserId] AND \na.[PlantId] = ugr.[PlantId]\nLEFT JOIN [Config].[UserGroup] as ug\nON ugr.[PlantId] = ug.[PlantId] AND\nugr.[UserGroupId] = ug.[UserGroupId]\n\nORDER BY a.[PlantId]\n--WHERE a.[PlantId] = '<A>'"
        # "Only Admin.Users checked"
        # "Only DB Column Names \nupdated to MCListbox Col0"
        # "Order by 1st Primary KEY"
        # "# of DB Table Columns\nused as Row0 in MCListbox"
        # "SELECT Table & Column Information FROM DB\nSELECT * FROM DB"
        n187 = event-data() -> ()  [unwired: 1 in, 6 out]
        n188 = call "DB - Columns INFO.vi"("Refnum in"=w405, "DB.dbo.Table"="DB.Admin.Users", "error in (no error)"=w404) -> ("IDENTITY COLUMN"=→"IDENTITY COLUMN":string, "Refnum out"=w375:T10, "COLUMN_NAME"=w387:string[], "DATA_TYPE"=w386:string[], "PRECISION"=w362:string[], "error out"=w367:errorcluster)  [unwired: 4 in, 3 out]
        n189 = call "DB - Split DB.Schema.Table.vi"("DB.Schema.Table"="DB.Config.UserGroup") -> ("DB.Schema.Table"=w354:T12)  [unwired: 10 in]
        n190 = call "DB - Split DB.Schema.Table.vi"("DB.Schema.Table"="DB.Config.UserGroupRelation") -> ("DB.Schema.Table"=w356:T12)  [unwired: 10 in]
        n191 = call "DB - Split DB.Schema.Table.vi"("DB.Schema.Table"="DB.Config.TabUserAccess") -> ("DB.Schema.Table"=w369:T12)  [unwired: 10 in]
        n192 = call "DB - Split DB.Schema.Table.vi"("DB.Schema.Table"="DB.Config.UserStationAccess") -> ("DB.Schema.Table"=w368:T12)  [unwired: 10 in]
        n193 = call "DB - Split DB.Schema.Table.vi"("DB.Schema.Table"="DB.Admin.Users") -> ("DB.Schema.Table"=w370:T12)  [unwired: 10 in]
        n194 = call "DB - Replace DB.Schema.Table.vi"("DB.Schema.Table 4"=w356, "DB.Schema.Table 3"=w368, "DB.Schema.Table 5"=w354, "DB.Schema.Table 2"=w369, "DB.Schema.Table"=w370, "string in"=w379) -> ("error out"=w377:errorcluster, "string out"=w378:string)  [unwired: 4 in]
        n195 = disable-structure shown="Disabled" {
          disable-tunnel: w378 -> [w455 w457]
          disable-tunnel: [w454 w457] -> w353
          disable-tunnel: w377 -> [w453 _]
          frame Disabled {
            # "PlantId"
            n196 = Search and Replace String(input string=w455, search string="<A>", error in=w453) -> (result string=w454:string)  [unwired: 5 in, 3 out]
          }
          frame Enabled {
          }
        }
        n197 = call-poly <vilib>:"DB Tools Execute Query.vi"("error in (no error)"=w367, "SQL query"=w353, "connection reference"=w375) -> ("error out"=w385:errorcluster, "recordset reference"=w384:T13)  [unwired: 5 in]
        n198 = call-poly <vilib>:"DB Tools Fetch Recordset Data.vi"("error in (no error)"=w385, "recordset reference"=w384) -> ("error out"=w380:errorcluster, "recordset data"=w383:variant[][], "recordset reference out"=w381:T13)  [unwired: 3 in]
        n199 = xnode "Database Variant To Data"("database variant"=w383, "type"=string[][] []) -> ("data"=w376:string[][])  [unwired: 1 in, 1 out]
        n200 = call-poly <vilib>:"DB Tools Free Object.vi"("error in (no error)"=w380, "recordset reference"=w381) -> ("error out"=w366:errorcluster, "connection reference"=w374:T10)  [unwired: 8 in]
        n201 = for {
          tunnel: w376 -> [w511]
          tunnel: w350 -> [w505] mode=indexing
          tunnel: [w510] -> w352 mode=indexing
          tunnel: w387 -> [w509]
          tunnel: w386 -> [w508]
          tunnel: w362 -> [w507]
          tunnel: [w503] -> w349 mode=indexing
          tunnel: [w502] -> w348 mode=indexing
          # "ColName"
          # "Column Number"
          n202 = Format Into String(w505) -> (resulting string=w506:string)  [unwired: 3 in, 1 out]
          n203 = Index Array(array=w511, index (col)=w505) -> (element=w510:string[])  [unwired: 1 in]
          n204 = Search 1D Array "Match Col Hdrs[]\nData Type"(1D array=w509, element=w506) -> (index of element=w504:i32)  [unwired: 1 in]
          n205 = Index Array(array=w508, index=w504) -> (element=w503:string)
          n206 = Index Array(array=w507, index=w504) -> (element=w502:string)
        }
        "Col Hdrs[] DB Data Type" <- w349
        "Col Hdrs[] DB Precision" <- w348
        n207 = local write "SQL Query"(w353) -> ()
        n208 = call "DB - Get Keys.vi"("error in (no error)"=w366, "DB.Schema.Table"="DB.Admin.Users", "Refnum in"=w374) -> ("error out"=w410:errorcluster, "Foreign Keys"=→"Foreign Keys":string[], "Primary Key"=w402:string[], "Refnum out"=w411:T10)  [unwired: 5 in]
        "Primary Keys" <- w402
        n209 = call "DB - Count.vi"("Include Inactive"="Include Inactive", "error in (no error)"=w410, "DB.dbo.Table"="DB.Admin.Users", "Refnum in"=w411) -> ("error out"=w400:errorcluster, "COUNT"=w399:i32)  [unwired: 5 in, 1 out]
        n210 = Index Array(array=w402) -> (element=w398:string)  [unwired: 1 in]
        "1st Primary KEY" <- w398
        n211 = local write "Record Count"(w399) -> ()
        n212 = Transpose 2D Array(2D array=w352) -> (transposed array=w351:string[][])
        "transposed array" <- w351
        n213 = String Length(string=w398) -> (length=w397:i32)
        n214 = Equal To 0? "Records=0"(x=w399) -> (x = 0?=w395:bool)
        n215 = Equal To 0? "PrimaryKey=0"(x=w397) -> (x = 0?=w396:bool)
        n216 = Or(x=w396, y=w395) -> (x .or. y?=w394:bool)
        n217 = for "Convert DB Data Type to Strings" {
          tunnel: w351 -> [w439] mode=indexing
          tunnel: w349 -> [w438]
          tunnel: [w437] -> w361 mode=indexing
          # "Row"
          n218 = for {
            tunnel: w439 -> [w441] mode=indexing
            tunnel: w438 -> [w442] mode=indexing
            tunnel: [w440] -> w437 mode=indexing
            # "Column"
            n219 = case shown="\"False\", Default" w442 {
              tunnel: w441 -> [w443 w445 w449]
              tunnel: [w443 w444 w448] -> w440
              frame "False", Default {
              }
              frame "bit" {
                n220 = case shown="\"0\"" w445 {
                  selector: w445 -> [_ w447]
                  tunnel: ["1" w447] -> w444
                  frame "-1", Default {
                  }
                  frame "0" {
                  }
                }
              }
              frame "datetime", "datetime2" {
                # "SQL Server Default"
                n221 = Equal?(x=w449, y="1900-01-01") -> (x = y?=w451:bool)
                n222 = Select(t="", s=w451, f=w449) -> (s? t:f=w448:string)
              }
            }
          }
        }
        n223 = case shown="False" w394 {
          tunnel: w400 -> [w519 w522]
          tunnel: [w518 w522] -> w390
          frame False {
            # "Record Updated Here"
            n224 = property on="Current Record" class="DigNum (strict)"(error in=w519, "Val(Sgnl)"=1) -> (error out=w518:errorcluster)  [unwired: 1 in, 1 out]
          }
          frame True {
            # "No Primary KEY\nor No Records"
            n225 = local write "Current Record"(0 ("Current Record")) -> ()
          }
        }
        "Property Node" <- w390
        n226 = local read "CellBG Unused Cells"() -> (w358:u32)
        n227 = local read "CellBG ColHdrs"() -> (w360:u32)
        n228 = local read "CellBG New Cells"() -> (w359:u32)
        n229 = Index Array(array=w361, index (col)=0 ("disabled index (col)")) -> (element=w364:string[])  [unwired: 1 in]
        n230 = property on="Property Node" class="MCListbox (strict)"(reference=w413, error in=w390, "ItemNames"=w361, "ActiveCell"=w417, "CellBG"=w358, "CellFontBold"=FALSE ("Active Cell:Cell Font:Bold"), "NumCols"="# of Columns", "NumRows"="# of Rows") -> (reference out=w409:refnum<vi>, error out=w408:errorcluster)
        n231 = property on="Search User ID" class="CmbBox (strict)"("Strings[]"=w364) -> ()  [unwired: 2 in, 2 out]
        n232 = property on="Property Node" class="MCListbox (strict)"(reference=w409, error in=w408, "ActiveCell"=w406, "CellBG"=w360) -> (reference out=w389:refnum<vi>, error out=w407:errorcluster)
        n233 = for {
          N: 0 -> [_]
          tunnel: w359 -> [w525]
          shift-right: [w529] -> w416
          shift-left: w407 -> [w530]
          shift-right: [w523] -> w415
          shift-left: w389 -> [w524]
          i -> [w528]
          # "Color Each Row"
          n234 = Bundle(w528, -2) -> (w526:cluster{i32, i32})  [unwired: 1 in]
          n235 = property on="Property Node" class="MCListbox (strict)"(reference=w524, error in=w530, "ActiveCell"=w526, "CellBG"=w525) -> (reference out=w523:refnum<vi>, error out=w529:errorcluster)
        }
        n236 = disable-structure shown="Enabled" {
          disable-tunnel: w416 -> [w424 w435]
          disable-tunnel: w415 -> [w422 w436]
          disable-tunnel: "# of Columns" -> [w421 _]
          disable-tunnel: [w420 w435] -> w392
          disable-tunnel: [w419 w436] -> w391
          disable-tunnel: w358 -> [w418 _]
          frame Disabled {
            n237 = for {
              N: 10 -> [_]
              tunnel: w418 -> [w430]
              tunnel: w421 -> [w428]
              shift-right: [w433] -> w420
              shift-left: w424 -> [w434]
              shift-right: [w425] -> w419
              shift-left: w422 -> [w426]
              i -> [w429]
              # "Invalid Leftover Columns"
              n238 = Add(x=w428, y=w429) -> (x+y=w427:i32)
              n239 = Bundle(-2, w427) -> (w432:cluster{i32, i32})  [unwired: 1 in]
              n240 = property on="Property Node" class="MCListbox (strict)"(reference=w426, error in=w434, "ActiveCell"=w432, "CellBG"=w430) -> (reference out=w425:refnum<vi>, error out=w433:errorcluster)
            }
          }
          frame Enabled {
          }
        }
        n241 = case shown="Error" w392 {
          tunnel: w391 -> [_ w517]
          frame No Error {
            n242 = property on="New" class="Bool"("DisabledEnum"=T6."Enabled" ("Disabled")) -> ()  [unwired: 2 in, 2 out]
          }
          frame Error {
            w514 = T6."Disabled and Grayed Out" ("Disabled")
            n243 = property on="Property Node" class="MCListbox (strict)"(reference=w517, "Value"=-1, "ItemNames"=string[][] [] ("Item Names")) -> (error out=w513:errorcluster)  [unwired: 1 in, 1 out]
            n244 = local write "Property Node"(w513) -> ()
            n245 = property on="Save" class="Bool"("DisabledEnum"=w514) -> ()  [unwired: 2 in, 2 out]
            n246 = property on="New" class="Bool"("DisabledEnum"=w514) -> ()  [unwired: 2 in, 2 out]
          }
        }
      }
      event Value Change {
        n247 = event-data() -> ("NewVal"=w533:T2)  [unwired: 1 in, 5 out]
        n248 = property class="MCListbox (strict)"(reference=w537) -> (error out=w531:errorcluster, "ItemNames"=w536:string[][])  [unwired: 1 in, 1 out]
        n249 = Index Array(array=w536, index (col)=0 ("disabled index (col)")) -> (element=w534:string[])  [unwired: 1 in]
        n250 = Search 1D Array(1D array=w534, element=w533) -> (index of element=w532:i32)  [unwired: 1 in]
        n251 = case shown="0, Default" w532 {
          tunnel: w532 -> [w540 _]
          tunnel: w531 -> [w538 _]
          frame 0, Default {
            # "Show Searched Row as Top Row"
            # "Leave 5 Rows on top"
            n252 = Subtract(x=w540, y=5) -> (x-y=w542:i32)
            n253 = Greater Or Equal To 0?(x=w542) -> (x >= 0?=w543:bool)
            n254 = Select(t=w542, s=w543, f=0) -> ()  [unwired: 1 out]
            n255 = Bundle("index of element"=w540, 0) -> (w544:cluster{"index of element":i32, i32})  [unwired: 1 in]
            n256 = property on="Multicolumn Listbox" class="MCListbox (strict)"(error in=w538, "Val(Sgnl)"=w540, "TopLeft"=w544) -> (error out=w539:errorcluster)  [unwired: 1 in, 1 out]
            n257 = local write "Property Node"(w539) -> ()
          }
          frame -1 {
          }
        }
      }
      event "Current Record": Value Change {
        n258 = event-data() -> ()  [unwired: 1 in, 6 out]
        n259 = local read "Record Count"() -> (w551:i32)
        n260 = In Range and Coerce(upper limit=w551, x="Current Record", lower limit=1) -> (coerced(x)=w552:i32, In Range?=w548:bool)
        n261 = control-ref of="Current Record"() -> (w550:refnum<vi>)
        n262 = case shown="True" w548 {
          tunnel: w556 -> [w560 w562]
          tunnel: w552 -> [w558 w563]
          tunnel: [w560 w562] -> w555
          tunnel: w554 -> [_ _]
          tunnel: "Current Record" -> [_ _]
          tunnel: w550 -> [w559 w564]
          tunnel: [w557 w561] -> w547
          frame False {
            # "To fire an event again so\nthat the calling VIs gets notified\n\nIt may mean that the same record will \nbe fetched again"
            # "Coerce back to Record #"
            n263 = property class="DigNum (strict)"(reference=w559, "Val(Sgnl)"=w558) -> (error out=w557:errorcluster)  [unwired: 1 in, 1 out]
          }
          frame True {
            # "Valid Record#"
            n264 = property class="DigNum (strict)"(reference=w564, "Value"=w563) -> (error out=w561:errorcluster)  [unwired: 1 in, 1 out]
          }
        }
        n265 = local write "Property Node"(w547) -> ()
      }
      event "Multicolumn Listbox": Value Change {
        # "USER Clicks on MCListbox\nDisable Save, Updates Details Header Cluster, Update Flags"
        n266 = event-data() -> ("Time"=→"MCListBox":u32, "NewVal"=w566:i32)  [unwired: 1 in, 4 out]
        "NewVal" <- w566
        n267 = property on="Save" class="Bool"("DisabledEnum"=T6."Disabled and Grayed Out" ("Disabled")) -> ()  [unwired: 2 in, 2 out]
        n268 = case shown="0, Default" w566 {
          selector: w566 -> [w569 _]
          frame 0, Default {
            w580 = ""
            # "Initially was just to call the EVENT Change but that will make SAVE Enabled\nSo now we call this section locally here."
            n269 = local read "New Record in UI not in DB"() -> (w570:bool)
            n270 = case shown="True" w570 {
              frame False {
                # "Current Record Count is correct"
              }
              frame True {
                # "Current Record Count must -1 since New Record\nno longer available and NOT in DB"
                n271 = local read "Record Count"() -> (w587:i32)
                n272 = local write "New Record in UI not in DB"(FALSE ("New Record in UI not in DB")) -> ()
                n273 = Decrement(x=w587) -> (x-1=w586:i32)
                n274 = local write "Record Count"(w586) -> ()
              }
            }
            n275 = Increment(x=w569) -> (x+1=w568:i32)
            n276 = local write "Current Record"(w568) -> ()
            n277 = property on="Password" class="Str"("Value"=w580) -> ()  [unwired: 2 in, 2 out]
            n278 = property on="Retype Password" class="Str"("Value"=w580) -> ()  [unwired: 2 in, 2 out]
            n279 = property on="User Details" class="Clust (strict)"() -> (error out=w578:errorcluster, "Controls[]"=w581:refnum<vi>[])  [unwired: 2 in, 1 out]
            n280 = for {
              tunnel: w581 -> [w606] mode=indexing
              tunnel: w569 -> [w595]
              tunnel: [w599] -> w579
              tunnel: w578 -> [w597]
              n281 = property on="Multicolumn Listbox" class="MCListbox (strict)"() -> ("ColHdrString"=w605:string[], "ItemNames"=w596:string[][])  [unwired: 2 in, 2 out]
              n282 = Index Array(array=w596, index (row)=w595, index (col)=0 ("disabled index (col)")) -> (element=w593:string)
              n283 = property on="Search User ID" class="CmbBox (strict)"("Value"=w593) -> ()  [unwired: 2 in, 2 out]
              n284 = property class="Ctl"(reference=w606, error in=w597) -> (reference out=w600:refnum<vi>, error out=w598:errorcluster, "Label.Text"=w604:string)
              n285 = local read "Col Hdrs[] DB Data Type"() -> (w601:string[])
              n286 = Search 1D Array(1D array=w605, element=w604) -> (index of element=w602:i32)  [unwired: 1 in]
              n287 = Greater Or Equal To 0?(x=w602) -> (x >= 0?=w603:bool)
              n288 = case shown="True" w603 {
                tunnel: w596 -> [_ w618]
                tunnel: w595 -> [_ w617]
                tunnel: w602 -> [_ w615]
                tunnel: w601 -> [_ w616]
                tunnel: w600 -> [_ w613]
                tunnel: [w607 w610] -> w599
                tunnel: w598 -> [w607 w609]
                frame False {
                }
                frame True {
                  # "Not used"
                  n289 = Index Array(array=w618, index (row)=w617, index (col)=w615) -> (element=w614:string)
                  n290 = Index Array(array=w616, index=w615) -> ()  [unwired: 1 out]
                  n291 = property class="Ctl"(reference=w613, error in=w609) -> (reference out=w611:refnum<vi>, error out=w608:errorcluster, "ClassName"=w612:string)
                  n292 = case shown="\"False\", Default" w612 {
                    tunnel: w614 -> [w621 w633 w640]
                    tunnel: w611 -> [w622 w627 w641]
                    tunnel: [w620 w624 w639] -> w610
                    tunnel: w608 -> [w619 w623 _]
                    frame "False", Default {
                      n293 = property class="Ctl"(reference=w622, error in=w619, "Value"=w621) -> (error out=w620:errorcluster)  [unwired: 1 out]
                    }
                    frame "Boolean" {
                      w628 = refnum<vi> refnum  # Boolean
                      n294 = Equal?(x="1", y=w633) -> (x = y?=w631:bool)
                      n295 = Select(t=TRUE, s=w631, f=FALSE) -> (s? t:f=w625:bool)
                      n296 = To More Specific Class(target class=w628, reference=w627) -> (specific class reference=w626:refnum<vi>)  [unwired: 1 in, 1 out]
                      n297 = property class="Bool"(reference=w626, error in=w623, "Value"=w625) -> (error out=w624:errorcluster)  [unwired: 1 out]
                    }
                    frame "AbsTime" {
                      w643 = refnum<vi> refnum  # AbsTime
                      n298 = call "String - Convert Str (YYYY-mm-dd HHcMMcSS) to TimeStamp.vi"("YYYY-mm-dd HH:MM:SS (String)"=w640) -> ("time stamp"=w635:timestamp)  [unwired: 9 in, 1 out]
                      n299 = To More Specific Class(target class=w643, reference=w641) -> (specific class reference=w642:refnum<vi>)  [unwired: 1 in, 1 out]
                      n300 = Greater?(x=w635, y=timestamp(31593600 s since 1904-01-01)) -> (0:w637:bool)
                      n301 = Select(t=w635, s=w637, f=timestamp(0 s since 1904-01-01) ("time stamp")) -> (s? t:f=w634:timestamp)
                      n302 = property class="AbsTime"(reference=w642, "Value"=w634) -> (error out=w639:errorcluster)  [unwired: 1 in, 1 out]
                    }
                  }
                }
              }
            }
            n303 = property on="Domain ID" class="CmbBox (strict)"(error in=w579) -> (error out=w571:errorcluster, "Value"=w572:T2)  [unwired: 1 in, 1 out]
            n304 = To Upper Case(1:w572) -> (0:w576:T2)
            n305 = Equal?(x=w576, y="LOCAL") -> (x = y?=w575:bool)
            n306 = case shown="False" w575 {
              tunnel: [u32 16777216 u32 16777215] -> w574
              tunnel: [T6."Disabled" ("Disabled") T6."Enabled" ("Disabled")] -> w573
              frame False {
                n307 = disable-structure shown="Disabled" {
                  frame Disabled {
                    w590 = TRUE
                    n308 = local write "Password Count Valid"(w590) -> ()
                    n309 = local write "Password Matched"(w590) -> ()
                  }
                  frame Enabled {
                  }
                }
              }
              frame True {
              }
            }
            n310 = local write "Property Node"(w571) -> ()
            n311 = disable-structure shown="Disabled" {
              disable-tunnel: w574 -> [w584 _]
              disable-tunnel: w573 -> [w583 _]
              frame Disabled {
                n312 = property on="User Name" class="Str"("Text.BGColor"=w584, "DisabledEnum"=w583) -> ()  [unwired: 2 in, 2 out]
              }
              frame Enabled {
              }
            }
            n313 = property on="Password" class="Str"("Text.BGColor"=w574, "DisabledEnum"=w573) -> ()  [unwired: 2 in, 2 out]
            n314 = property on="Retype Password" class="Str"("Text.BGColor"=w574, "DisabledEnum"=w573) -> ()  [unwired: 2 in, 2 out]
            n315 = flat-sequence "Save Flags" {
              frame #0 {
                w582 = TRUE
                # "Since records exsiting, assume all already valid\nThey will be checked again when user edits that\nparticular field.\nThey will be cleared when New Record is pressed"
                n316 = local write "All Mandatory Fields Filled"(w582) -> ()
                n317 = local write "Email Valid"(w582) -> ()
                n318 = local write "Password Count Valid"(w582) -> ()
                n319 = local write "Password Matched"(w582) -> ()
              }
            }
          }
          frame -1 {
            n320 = property on="Search User ID" class="CmbBox (strict)"("Value"="") -> ()  [unwired: 2 in, 2 out]
            n321 = property on="Save" class="Bool"("DisabledEnum"=T6."Disabled and Grayed Out" ("Disabled")) -> ()  [unwired: 2 in, 2 out]
          }
        }
      }
      event "Multicolumn Listbox": Mouse Up {
        # "Mouse Up seems to work BEST for Sorting"
        n322 = event-data() -> ("CtlRef"=w649:refnum<vi>)  [unwired: 1 in, 7 out]
        n323 = control-ref of="Ascending"() -> (w648:refnum<vi>)
        n324 = call "MCListbox Event - Sort Table.vi"("Clicked Color"=u32 16777216, "Sort Order Boolean Ref"=w648, "MCListBox Ref"=w649) -> ("ItemNames"=w651:string[][])  [unwired: 8 in]
        n325 = Index Array(array=w651, index (col)=0 ("disabled index (col)")) -> (element=w647:string[])  [unwired: 1 in]
        n326 = Array Size(array=w647) -> (size(s)=w646:i32)
        n327 = case shown="1, Default" w646 {
          tunnel: w647 -> [_ w653]
          frame 0 {
          }
          frame 1, Default {
            n328 = property on="Search User ID" class="CmbBox (strict)"("Strings[]"=w653) -> ()  [unwired: 2 in, 2 out]
          }
        }
      }
      event "------------------------------------        User Details Header EVENTS     ------------------------------------": Value Change {
        # "DUMMY EVENT"
        n329 = event-data() -> ()  [unwired: 1 in, 6 out]
      }
      event Mouse Down? {
        # "TabAccessId, StationAccessId, UserGroupID\nThe  respective Description (if applicable) will be update at its\nEVENT CHANGE"
        # "Query for Values of [PlantId] OR[TabAccessId] OR [StationAccessId] OR [DomainId] OR  [UserGroupId] \nto populate their respective ComboBox"
        n330 = event-data() -> ("CtlRef"=w669:refnum<vi>)  [unwired: 1 in, 7 out]
        n331 = property class="CmbBox (strict)"(reference=w669) -> ("Label.Text"=w667:string)  [unwired: 1 in, 2 out]
        n332 = property on="Plant ID" class="CmbBox (strict)"() -> ("Value"=w655:T2)  [unwired: 2 in, 2 out]
        n333 = Search 1D Array(1D array=w668, element=w667) -> (index of element=w666:i32)  [unwired: 1 in]
        n334 = Index Array(array=w665, index=w666) -> (element=w664:T7)
        n335 = Format Into String(w664) -> (resulting string=w658:string)  [unwired: 3 in, 1 out]
        n336 = case shown="\"PlantId\"" w658 {
          tunnel: [w684 w685 w688 "DB.Config.Domain" "DB.Config.Plant"] -> w657
          tunnel: ["USE [<DB>]\n\nSELECT [<A>]\nFROM [<Schema>].[<Table>]\n\nWHERE [PlantID] = '<B>' AND [Inactive] = '0'\nGROUP BY [<A>]\n" "USE [<DB>]\n\nSELECT [<A>]\nFROM [<Schema>].[<Table>]\n\nWHERE [PlantID] = '<B>' AND [Inactive] = '0'\nGROUP BY [<A>]\n" "USE [<DB>]\n\nSELECT [<A>]\nFROM [<Schema>].[<Table>]\n\nWHERE [PlantID] = '<B>' AND [Inactive] = '0'\nGROUP BY [<A>]\n" "USE [<DB>]\n\nSELECT [<A>]\nFROM [<Schema>].[<Table>]\n\nWHERE [Inactive] = '0'\nGROUP BY [<A>]\n" "USE [<DB>]\n\nSELECT [<A>]\nFROM [<Schema>].[<Table>]\n\nWHERE [Inactive] = '0'\nGROUP BY [<A>]\n"] -> w656
          frame "StationAccessId", Default {
            n337 = local read "DB.Config.UserStationAccess"() -> (w684:string)
          }
          frame "UserGroupId" {
            n338 = local read "DB.Config.UserGroup"() -> (w685:string)
          }
          frame "TabAccessId" {
            n339 = local read "DB.Config.TabUserAccess"() -> (w688:string)
          }
          frame "DomainId" {
            # "No [PlantId] in Config.Domain"
          }
          frame "PlantId" {
          }
        }
        n340 = call "DB - Split DB.Schema.Table.vi"("DB.Schema.Table"=w657) -> ("DB.Schema.Table"=w675:T12)  [unwired: 10 in]
        n341 = call "DB - Replace DB.Schema.Table.vi"("DB.Schema.Table"=w675, "string in"=w656) -> ("string out"=w663:string)  [unwired: 8 in, 1 out]
        n342 = Search and Replace String(replace all?=TRUE ("replace all? (F)"), input string=w663, search string="<A>", replace string=w658) -> (result string=w662:string)  [unwired: 4 in, 3 out]
        n343 = Search and Replace String(input string=w662, search string="<B>", replace string=w655) -> (result string=w661:string)  [unwired: 5 in, 3 out]
        n344 = call-poly <vilib>:"DB Tools Execute Query.vi"("SQL query"=w661, "connection reference"=w676) -> ("error out"=w682:errorcluster, "recordset reference"=w681:T13)  [unwired: 6 in]
        n345 = call-poly <vilib>:"DB Tools Fetch Recordset Data.vi"("error in (no error)"=w682, "recordset reference"=w681) -> ("error out"=w677:errorcluster, "recordset data"=w680:variant[][], "recordset reference out"=w678:T13)  [unwired: 3 in]
        n346 = xnode "Database Variant To Data"("database variant"=w680, "type"=string[][] []) -> ("data"=w673:string[][])  [unwired: 1 in, 1 out]
        n347 = call-poly <vilib>:"DB Tools Free Object.vi"("error in (no error)"=w677, "recordset reference"=w678) -> ("error out"=w654:errorcluster)  [unwired: 8 in, 1 out]
        n348 = Index Array(array=w673, index (col)=0 ("disabled index (col)")) -> (element=w671:string[])  [unwired: 1 in]
        n349 = local write "SQL Query"(w661) -> ()
        n350 = local write "DB"(w654) -> ()
        n351 = property class="CmbBox (strict)"(reference=w669, error in=w654, "Strings[]"=w671) -> (error out=w670:errorcluster)  [unwired: 1 out]
        n352 = local write "Property Node"(w670) -> ()
        n353 = event-data() -> ()  [unwired: 2 in, 1 out]
      }
      event Value Change {
        # "Query for Description of [TabAccessId] OR [StationAccessId]"
        n354 = event-data() -> ("CtlRef"=w770:refnum<vi>)  [unwired: 1 in, 5 out]
        n355 = property class="CmbBox (strict)"(reference=w770) -> ("Label.Text"=w768:string, "Value"=w740:T2)  [unwired: 1 in, 2 out]
        n356 = Search 1D Array(1D array=w769, element=w768) -> (index of element=w767:i32)  [unwired: 1 in]
        n357 = Index Array(array=w766, index=w767) -> (element=w765:T7)
        n358 = Format Into String "[Column Name]"(w765) -> (resulting string=w741:string)  [unwired: 3 in, 1 out]
        n359 = case shown="\"UserGroupId\"" w741 {
          tunnel: [w772 w774 w775] -> w746
          tunnel: [w771 w773 w776] -> w739
          frame "StationAccessId", Default {
            n360 = local read "DB.Config.UserStationAccess"() -> (w772:string)
            n361 = control-ref of="Station Access"() -> (w771:refnum<vi>)
          }
          frame "TabAccessId" {
            n362 = local read "DB.Config.TabUserAccess"() -> (w774:string)
            n363 = control-ref of="Tab Access"() -> (w773:refnum<vi>)
          }
          frame "UserGroupId" {
            n364 = local read "DB.Config.UserGroup"() -> (w775:string)
            n365 = control-ref of="User Group"() -> (w776:refnum<vi>)
          }
        }
        n366 = call "DB - Split DB.Schema.Table.vi"("DB.Schema.Table"=w746) -> ("DB.Schema.Table"=w757:T12)  [unwired: 10 in]
        n367 = call "DB - Replace DB.Schema.Table.vi"("DB.Schema.Table"=w757, "string in"="USE [<DB>]\n\nSELECT [Description]\nFROM [<Schema>].[<Table>]\n\nWHERE [<A>] = '<B>' AND [PlantID] = '<C>' AND [Inactive] = '0'\n\n") -> ("string out"=w750:string)  [unwired: 8 in, 1 out]
        n368 = Search and Replace String(replace all?=TRUE ("replace all? (F)"), input string=w750, search string="<A>", replace string=w741) -> (result string=w749:string)  [unwired: 4 in, 3 out]
        n369 = Search and Replace String(input string=w749, search string="<B>", replace string=w740) -> (result string=w744:string)  [unwired: 5 in, 3 out]
        n370 = property on="Plant ID" class="CmbBox (strict)"() -> ("Value"=w737:T2)  [unwired: 2 in, 2 out]
        n371 = Search and Replace String(input string=w744, search string="<C>", replace string=w737) -> (result string=w743:string)  [unwired: 5 in, 3 out]
        n372 = call-poly <vilib>:"DB Tools Execute Query.vi"("SQL query"=w743, "connection reference"=w745) -> ("error out"=w764:errorcluster, "recordset reference"=w763:T13)  [unwired: 6 in]
        n373 = call-poly <vilib>:"DB Tools Fetch Recordset Data.vi"("error in (no error)"=w764, "recordset reference"=w763) -> ("error out"=w759:errorcluster, "recordset data"=w762:variant[][], "recordset reference out"=w760:T13)  [unwired: 3 in]
        n374 = xnode "Database Variant To Data"("database variant"=w762, "type"=string[][] []) -> ("data"=w755:string[][])  [unwired: 1 in, 1 out]
        n375 = call-poly <vilib>:"DB Tools Free Object.vi"("error in (no error)"=w759, "recordset reference"=w760) -> ("error out"=w751:errorcluster)  [unwired: 8 in, 1 out]
        n376 = Index Array(array=w755, index (row)=0 ("disabled index (row)"), index (col)=0 ("disabled index (col)")) -> (element=w753:string)
        n377 = local write "DB"(w751) -> ()
        n378 = local write "SQL Query"(w743) -> ()
        n379 = property class="Str"(reference=w739, error in=w751, "Value"=w753) -> (error out=w752:errorcluster)  [unwired: 1 out]
        n380 = local write "Property Node"(w752) -> ()
      }
      event Value Change {
        # "Enabled User Name, Password and Reenter Password Controls"
        n381 = event-data() -> ("NewVal"=w826:T2)  [unwired: 1 in, 5 out]
        n382 = To Upper Case(1:w826) -> (0:w825:T2)
        n383 = Equal?(x=w825, y="LOCAL") -> (x = y?=w824:bool)
        n384 = case shown="False" w824 {
          tunnel: [u32 16777216 u32 16777215] -> w823
          tunnel: [T6."Disabled" ("Disabled") T6."Enabled" ("Disabled")] -> w822
          frame False {
            w831 = TRUE
            n385 = local write "Password Count Valid"(w831) -> ()
            n386 = local write "Password Matched"(w831) -> ()
          }
          frame True {
          }
        }
        n387 = disable-structure shown="Disabled" {
          disable-tunnel: w823 -> [w830 _]
          disable-tunnel: w822 -> [w829 _]
          disable-tunnel: "" -> [w828 _]
          frame Disabled {
            n388 = property on="User Name" class="Str"("Text.BGColor"=w830, "DisabledEnum"=w829, "Value"=w828) -> ()  [unwired: 2 in, 2 out]
          }
          frame Enabled {
          }
        }
        n389 = property on="Password" class="Str"("Text.BGColor"=w823, "DisabledEnum"=w822) -> ()  [unwired: 2 in, 2 out]
        n390 = property on="Retype Password" class="Str"("Text.BGColor"=w823, "DisabledEnum"=w822) -> ()  [unwired: 2 in, 2 out]
      }
      event "User Details.User ID": Key Down {
        n391 = event-data() -> ("VKey"=w836:T14)  [unwired: 1 in, 9 out]
        n392 = case shown="\"Enter\", \"Return\"" w836 {
          frame "ASCII", Default {
          }
          frame "Enter", "Return" {
            n393 = property on="Domain ID" class="CmbBox (strict)"() -> ("Value"=w843:T2)  [unwired: 2 in, 2 out]
            n394 = property on="User ID" class="Str"() -> ("Value"=w842:string)  [unwired: 2 in, 2 out]
            n395 = call "Logon - Module.vi"("Logon - Enum"=Logon_-_Enum."Check AD", "Domain"=w843, "Logon User"=w842) -> ("Error Out"=→"Logon":errorcluster, "AD Info"=w840:T15)  [unwired: 3 in, 4 out]
            n396 = Unbundle By Name(w840) -> ("Logon Full Name"=w837:string, "AD available"=w839:bool)
            n397 = property on="User Name" class="Str"("Value"=w837) -> ()  [unwired: 2 in, 2 out]
            n398 = case shown="True" w839 {
              tunnel: w837 -> [_ w850]
              frame False {
                # "AD not available"
                n399 = property on="Domain ID" class="CmbBox (strict)"("Value"="Local") -> ()  [unwired: 2 in, 2 out]
                n400 = local read "Application"() -> (w844:string)
                n401 = call "Msgbox - Message Handler.vi"("Application (Default SRTRS)"=w844, "Short Description (When DB Not Available)"="Domain Not Available", "Description (When DB Not Available)"="Cameron domain not available. Please confirm domain availability before retry.", "<.?....> Message Code"="<E 602>" ("Short Description (When DB Not Available)")) -> ("MHandler Error"=w846:errorcluster)  [unwired: 5 in, 2 out]
                n402 = local write "MHandler"(w846) -> ()
              }
              frame True {
                # "AD available"
                n403 = case shown="\"\"" w850 {
                  frame "" {
                    # "No Name found"
                    n404 = local read "Application"() -> (w851:string)
                    n405 = call "Msgbox - Message Handler.vi"("Application (Default SRTRS)"=w851, "Short Description (When DB Not Available)"="Invalid Domain User", "Description (When DB Not Available)"="User ID entered not available in Cameron Domain.", "<.?....> Message Code"="<E 603>") -> ("MHandler Error"=w855:errorcluster)  [unwired: 5 in, 2 out]
                    n406 = local write "MHandler"(w855) -> ()
                  }
                  frame "True", Default {
                  }
                }
              }
            }
          }
        }
      }
      event "User Details": Value Change {
        w866 = string[] ["Password", "Retype Password"]  # Mandatory Fields
        w867 = string[] ["User ID", "User Name", "SAP No.", "Mobile", "Email", "Tab Access ID", "Station Access ID", "Plant ID", "Domain ID"]  # Mandatory Fields
        # "Any Changes in Cluster will fire this event. However we cannot detect which Control in the Cluster has changed. \nEach Control in the Cluster must have their own EVENT Change if we want to process that EVENT individually\nSet Save to Enabled if All mandatory Fields filled"
        n407 = event-data() -> ("Time"=→"User Details 2":u32, "CtlRef"=w876:refnum<vi>)  [unwired: 1 in, 4 out]
        n408 = property on="Domain ID" class="CmbBox (strict)"() -> ("Value"=w869:T2)  [unwired: 2 in, 2 out]
        n409 = Equal?(x=w869, y="Local") -> (x = y?=w862:bool)
        n410 = property on="Property Node" class="MCListbox (strict)"(reference=w875) -> ("Value"=w874:i32)  [unwired: 1 in, 2 out]
        n411 = control-ref of="User Details"() -> (w872:refnum<vi>)
        n412 = Select(t=w866, s=w862, f=string[] []) -> (s? t:f=w864:string[])
        n413 = property class="Clust (strict)"(reference=w872) -> ("Controls[]"=w871:refnum<vi>[])  [unwired: 1 in, 2 out]
        n414 = Less Than 0?(x=w874) -> (x < 0?=w873:bool)
        n415 = disable-structure shown="Disabled" {
          disable-tunnel: w876 -> [w916 _]
          frame Disabled {
            w914 = string[] ["User ID", "User Name", "SAP No.", "Tab Access", "Station Access", "Inactive", "Mobile", "Email", "Tab Access ID", "Station Access ID", "Plant ID"]  # Madatory Field
            n416 = property class="Clust (strict)"(reference=w916) -> ("Controls[]"=w915:refnum<vi>[])  [unwired: 1 in, 2 out]
            n417 = for {
              tunnel: w915 -> [w921] mode=indexing
              tunnel: w914 -> [w919]
              n418 = property class="Ctl"(reference=w921) -> (reference out=w917:refnum<vi>, "Label.Text"=w920:string)  [unwired: 1 in, 1 out]
              n419 = Search 1D Array(1D array=w919, element=w920) -> (index of element=w918:i32)  [unwired: 1 in]
              n420 = case shown="0, Default" w918 {
                tunnel: w917 -> [_ _]
                frame 0, Default {
                }
                frame -1 {
                }
              }
            }
          }
          frame Enabled {
          }
        }
        n421 = Build Array (concatenate)(w867, w864) -> (w863:string[])
        n422 = case shown="True" w873 {
          frame False {
          }
          frame True {
            # "No Row Selected, Must be New Record"
            n423 = local read "New Record in UI not in DB"() -> (w922:bool)
            n424 = case shown="False" w922 {
              frame False {
                # "New Record NOT Flagged yet."
                n425 = local read "Record Count"() -> (w924:i32)
                n426 = local write "New Record in UI not in DB"(TRUE ("New Record in UI not in DB")) -> ()
                n427 = Increment(x=w924) -> (x+1=w923:i32)
                n428 = local write "Current Record"(w923) -> ()
                n429 = local write "Record Count"(w923) -> ()
              }
              frame True {
                # "New Record Flagged already\nProbably by NEW Button EVENT"
              }
            }
          }
        }
        n430 = for {
          tunnel: w871 -> [w898] mode=indexing
          tunnel: w863 -> [w896]
          tunnel: [w891] -> w870 mode=indexing
          tunnel: [w892] -> w858 mode=indexing if=w891
          n431 = property class="Ctl"(reference=w898) -> (reference out=w893:refnum<vi>, "Label.Text"=w897:string, "Value"=w894:variant)  [unwired: 1 in, 1 out]
          n432 = Search 1D Array(1D array=w896, element=w897) -> (index of element=w895:i32)  [unwired: 1 in]
          n433 = case shown="0, Default" w895 {
            tunnel: w894 -> [w905 _]
            tunnel: [w901 _] -> w891
            tunnel: w893 -> [w900 _]
            tunnel: [w899 _] -> w892
            frame 0, Default {
              # "Mandatory Fields"
              n434 = Variant To Data(type="", Variant=w905) -> (data=w903:string)  [unwired: 1 in, 1 out]
              n435 = String Length(string=w903) -> (length=w902:i32)
              n436 = case shown="0" w902 {
                tunnel: [TRUE _] -> w901
                tunnel: w900 -> [w908 _]
                tunnel: [w906 _] -> w899
                frame 0 {
                  # "Blank"
                  n437 = property class="Ctl"(reference=w908) -> ("Caption.InterpretAsUnicode"=w909:bool)  [unwired: 1 in, 2 out]
                  n438 = property class="Ctl"(reference=w908) -> ("Caption.Text"=w907:string)  [unwired: 1 in, 2 out]
                  n439 = case shown="False" w909 {
                    tunnel: w907 -> [w912 w913]
                    tunnel: [w911 w913] -> w906
                    frame False {
                      n440 = call "tool_Unicode_Convert ASCII to Unicode (Scalar).vi"("ASCII"=w912) -> ("Unicode"=w911:string)  [unwired: 4 in]
                    }
                    frame True {
                    }
                  }
                }
                frame 1, Default {
                }
              }
            }
            frame -1 {
            }
          }
        }
        "Controls (Caption) that are blank (Unicode)" <- w858
        n441 = case shown="True" w862 {
          tunnel: [FALSE w881] -> w861
          frame False {
          }
          frame True {
            # "Password must be at least 8 characters."
            # "Password MUST Match"
            n442 = property on="Password" class="Str"() -> ("Value"=w885:string)  [unwired: 2 in, 2 out]
            n443 = property on="Retype Password" class="Str"() -> ("Value"=w884:string)  [unwired: 2 in, 2 out]
            n444 = String Length(string=w884) -> (length=w883:i32)
            n445 = Equal?(x=w885, y=w884) -> (x = y?=w879:bool)
            "Password Matched" <- w879
            n446 = Greater Or Equal?(x=w883, y=8) -> (x >= y?=w880:bool)
            "Password Count Valid" <- w880
            n447 = And(x=w879, y=w880) -> (x .and. y?=w881:bool)
          }
        }
        n448 = Or Array Elements(Boolean array=w870) -> (logical OR=w857:bool)
        n449 = Not(x=w857) -> (.not. x?=w856:bool)
        "All Mandatory Fields Filled" <- w856
        n450 = And(x=w856, y=w861) -> (x .and. y?=w859:bool)
        n451 = case shown="False" w859 {
          tunnel: [T6."Enabled" ("Disabled") w888] -> w860
          frame False {
            # "Either Blank Mandatory Fields OR\nPassword MisMatch (if Local)"
          }
          frame True {
            # "No Blank Mandatory Field AND \nPassword OK (Local)"
            n452 = Select(t=T6."Disabled and Grayed Out" ("Disabled"), s="Save Enabled depends on \nFilled Mandatory Fields", f=T6."Enabled" ("Disabled")) -> (s? t:f=w888:T6)
          }
        }
        n453 = property on="Save" class="Bool"("DisabledEnum"=w860) -> ()  [unwired: 2 in, 2 out]
      }
      event "User Details.User ID", "User Details.User Name", "User Details.SAP No.", "User Details.Mobile", "User Details.Email", "User Details.Password", "User Details.Retype Password": Value Change {
        # "In this case, only Strings Controls are chosen, so the rest of the cases do not matter."
        # "CAST relevant Controls in Cluster to follow the DB's Length"
        n454 = event-data() -> ("CtlRef"=w932:refnum<vi>)  [unwired: 1 in, 5 out]
        n455 = property on="Property Node" class="MCListbox (strict)"(reference=w929) -> ("ColHdrString"=w931:string[])  [unwired: 1 in, 2 out]
        n456 = property class="Str"(reference=w932) -> (reference out=w933:refnum<vi>, error out=w927:errorcluster, "Label.Text"=w928:string, "ClassName"=w939:string, "Value"=w938:string)  [unwired: 1 in]
        n457 = local read "Col Hdrs[] DB Precision"() -> (w936:string[])
        n458 = local read "Col Hdrs[] DB Data Type"() -> (w937:string[])
        n459 = Search 1D Array "Index of Col Hdrs[]"(1D array=w931, element=w928) -> (index of element=w930:i32)  [unwired: 1 in]
        n460 = Index Array(array=w937, index=w930) -> (element=w935:string)
        n461 = Index Array(array=w936, index=w930) -> (element=w934:string)
        n462 = case shown="\"ComboBox\", \"String\"" w939 {
          tunnel: w938 -> [_ _ _ _]
          tunnel: [w954 w1024 "" w1042] -> _
          tunnel: w935 -> [w946 _ _ _]
          tunnel: w934 -> [w956 w1029 _ _]
          tunnel: w933 -> [w949 w1034 _ w1050]
          tunnel: w928 -> [w947 _ _ _]
          tunnel: w927 -> [w944 w1023 w1036 w1041]
          tunnel: [w940 w1021 w1036 w1038] -> w926
          frame "ComboBox", "String" {
            w950 = refnum<vi> refnum  # String
            # "ComboBox may be set to Disallow \"undefined Strings\"\nIf you want to Force to select only listed items in ComboBox"
            n463 = To More Specific Class(target class=w950, reference=w949, error in=w944) -> (specific class reference=w948:refnum<vi>, error out=w943:errorcluster)
            n464 = case "Special Cases" shown="\"Email\"" w947 {
              tunnel: w946 -> [w957 _ _]
              tunnel: [w957 "Numbers Only" "Email" ("String")] -> w945
              frame "False", Default {
              }
              frame "Mobile" {
                (unwired) "Numbers & Hyphen"
                # "Numbers Only"
              }
              frame "Email" {
              }
            }
            n465 = property class="Str"(reference=w948, error in=w943) -> (reference out=w955:refnum<vi>, error out=w942:errorcluster, "Value"=w953:string)
            n466 = Variant To Data(error in=w942, type="", Variant=w953) -> (data=w952:string, error out=w941:errorcluster)
            n467 = case shown="\"Email\"" w945 {
              tunnel: w952 -> [_ w966 w975 w979 w988 w1008 w1016]
              tunnel: w956 -> [_ _ _ _ w987 w1007 w1018]
              tunnel: w955 -> [_ w964 w973 _ w985 w1005 w1014]
              tunnel: [_ w963 w970 w978 w984 w992 w1011] -> w954
              tunnel: w941 -> [w960 w962 w969 w977 w983 w990 w1010]
              tunnel: [w960 w961 w968 w977 w982 w989 w1009] -> w940
              frame "False", Default {
                # "unknown"
              }
              frame "Numbers & Hyphen" {
                n468 = Search and Replace String(replace all?=TRUE ("replace all? (F)"), input string=w966, search string="[^0-9-]") -> (result string=w963:string)  [unwired: 5 in, 3 out]
                n469 = property class="Str"(reference=w964, error in=w962, "Value"=w963) -> (error out=w961:errorcluster)  [unwired: 1 out]
              }
              frame "Numbers Only" {
                # "Remove heading 0s"
                # "Keep numbers only"
                # "No 0s in front"
                n470 = Search and Replace String(replace all?=TRUE ("replace all? (F)"), input string=w975, search string="[^0-9]") -> (result string=w971:string)  [unwired: 5 in, 3 out]
                n471 = Search and Replace String(input string=w971, search string="^0+") -> (result string=w970:string)  [unwired: 6 in, 3 out]
                n472 = property class="Str"(reference=w973, error in=w969, "Value"=w970) -> (error out=w968:errorcluster)  [unwired: 1 out]
              }
              frame "bit" {
                n473 = case shown="\"False\", Default" w979 {
                  tunnel: ["0" "1"] -> w978
                  frame "False", Default {
                  }
                  frame "1", "T", "TRUE", "True" {
                  }
                }
              }
              frame "nvarchar", "varchar" {
                n474 = Decimal String To Number(string=w987) -> (number=w986:i32)  [unwired: 2 in, 1 out]
                n475 = Search/Split String(string=w988, offset (0)=w986) -> (substring before match=w984:string)  [unwired: 1 in, 2 out]
                n476 = property class="Str"(reference=w985, error in=w983, "Value"=w984) -> (error out=w982:errorcluster)  [unwired: 1 out]
              }
              frame "Email" {
                n477 = Decimal String To Number(string=w1007) -> (number=w1006:i32)  [unwired: 2 in, 1 out]
                n478 = Search/Split String(string=w1008, offset (0)=w1006) -> (substring before match=w992:string)  [unwired: 1 in, 2 out]
                n479 = property class="Str"(reference=w1005, error in=w990, "Value"=w992) -> (error out=w989:errorcluster)  [unwired: 1 out]
                n480 = Match Pattern(string=w992, regular expression="@") -> (before substring=w1003:string, after substring=w1002:string)  [unwired: 1 in, 2 out]
                n481 = String Length(string=w1003) -> (length=w996:i32)
                n482 = Match Pattern(string=w1002, regular expression="\\.") -> (before substring=w1000:string, after substring=w999:string)  [unwired: 1 in, 2 out]
                n483 = String Length(string=w1000) -> (length=w997:i32)
                n484 = String Length(string=w999) -> (length=w998:i32)
                n485 = Greater Than 0?(x=w996) -> (x > 0?=w995:bool)
                n486 = Greater Than 0?(x=w997) -> (x > 0?=w994:bool)
                n487 = Greater Than 0?(x=w998) -> (x > 0?=w993:bool)
                n488 = Compound Arithmetic op=AND(w995, w994, w993) -> (→"Email Valid":bool)
              }
              frame "int" {
                n489 = Decimal String To Number(string=w1018) -> (number=w1017:i32)  [unwired: 2 in, 1 out]
                n490 = Search/Split String(string=w1016, offset (0)=w1017) -> (substring before match=w1015:string)  [unwired: 1 in, 2 out]
                n491 = Decimal String To Number(string=w1015) -> (number=w1013:i32)  [unwired: 2 in, 1 out]
                n492 = Number To Decimal String(number=w1013, width (-)=i16 0) -> (decimal integer string=w1011:string)
                n493 = property class="Str"(reference=w1014, error in=w1010, "Value"=w1011) -> (error out=w1009:errorcluster)  [unwired: 1 out]
              }
            }
          }
          frame "Digital", "Numeric" {
            w1035 = refnum<vi> refnum  # Numeric
            n494 = To More Specific Class(target class=w1035, reference=w1034, error in=w1023) -> (specific class reference=w1033:refnum<vi>, error out=w1022:errorcluster)
            n495 = property class="Num"(reference=w1033, error in=w1022) -> (reference out=w1025:refnum<vi>, error out=w1020:errorcluster, "Value"=w1032:variant)
            n496 = Variant To Data(error in=w1020, type=0, Variant=w1032) -> (data=w1030:i32, error out=w1019:errorcluster)
            n497 = Format Into String(w1030) -> (resulting string=w1027:string)  [unwired: 3 in, 1 out]
            n498 = Decimal String To Number(string=w1029) -> (number=w1028:i32)  [unwired: 2 in, 1 out]
            n499 = Search/Split String(string=w1027, offset (0)=w1028) -> (substring before match=w1024:string)  [unwired: 1 in, 2 out]
            n500 = Decimal String To Number(string=w1024) -> (number=w1026:i32)  [unwired: 2 in, 1 out]
            n501 = property class="Num"(reference=w1025, error in=w1019, "Value"=w1026) -> (error out=w1021:errorcluster)  [unwired: 1 out]
          }
          frame Default {
          }
          frame "Boolean" {
            w1049 = refnum<vi> refnum  # Boolean
            n502 = To More Specific Class(target class=w1049, reference=w1050, error in=w1041) -> (specific class reference=w1048:refnum<vi>, error out=w1040:errorcluster)
            n503 = property class="Bool"(reference=w1048, error in=w1040) -> (error out=w1039:errorcluster, "Value"=w1043:variant)  [unwired: 1 out]
            n504 = Variant To Data(error in=w1039, type=TRUE, Variant=w1043) -> (data=w1046:bool, error out=w1038:errorcluster)
            n505 = Select(t="1", s=w1046, f="0") -> (s? t:f=w1042:string)
          }
        }
        n506 = local write "Property Node"(w926) -> ()
      }
      event "------------------------------------------        Unused EVENTS     ----------------------------------------": Value Change {
        # "EVENTS Not used in this VI"
        n507 = event-data() -> ()  [unwired: 1 in, 6 out]
      }
      event "Next Button", "Previous Button", "Last Button", "First Button", "Include Inactive": Value Change {
        # "NOT used in DB UI - Admin User"
        n508 = event-data() -> ("CtlRef"=w1051:refnum<vi>)  [unwired: 1 in, 5 out]
        n509 = disable-structure shown="Disabled" {
          disable-tunnel: [w1055 _] -> _
          disable-tunnel: w1053 -> [w1061 _]
          disable-tunnel: w1052 -> [w1060 _]
          disable-tunnel: w1051 -> [w1054 _]
          frame Disabled {
            n510 = control-ref of="Include Inactive"() -> (w1056:refnum<vi>)
            n511 = local read "New Record in UI not in DB"() -> (w1058:bool)
            n512 = Equal?(x=w1054, y=w1056) -> (x = y?=w1055:bool)
            n513 = case shown="True" w1058 {
              tunnel: [_ errorcluster {"status"=FALSE, "code"=0, "source"=""} ("error constant")] -> w1057
              frame False {
              }
              frame True {
                n514 = local read "Record Count"() -> (w1073:i32)
                n515 = local write "New Record in UI not in DB"(FALSE ("New Record in UI not in DB")) -> ()
                n516 = Decrement(x=w1073) -> (x-1=w1072:i32)
                n517 = local write "Record Count"(w1072) -> ()
              }
            }
            n518 = Build Array("First Button", "Previous Button", "Next Button", "Last Button", w1055) -> (w1066:bool[])
            n519 = Search 1D Array(1D array=w1066, element=TRUE) -> (index of element=w1059:i32)  [unwired: 1 in]
            n520 = property on="Current Record" class="DigNum (strict)"() -> ("Value"=w1070:i32)  [unwired: 2 in, 2 out]
            n521 = case shown="4" w1059 {
              tunnel: w1070 -> [_ w1078 w1080 _ w1082]
              tunnel: [1 w1077 w1079 w1081 w1082] -> w1069
              tunnel: w1061 -> [_ _ _ _ _]
              tunnel: w1060 -> [_ _ _ _ _]
              tunnel: w1057 -> [_ _ _ _ _]
              frame 0, Default {
                # "1st Record"
              }
              frame 1 {
                # "Previous"
                n522 = Decrement(x=w1078) -> (x-1=w1077:i32)
              }
              frame 2 {
                # "Next"
                n523 = Increment(x=w1080) -> (x+1=w1079:i32)
              }
              frame 3 {
                # "Last Record"
                n524 = local read "Record Count"() -> (w1081:i32)
              }
              frame 4 {
                # "Refresh the entireTable because we need to update # of Records also"
                # "Include Invalid"
                n525 = disable-structure shown="Disabled" {
                  frame Disabled {
                    n526 = property on="Property Node" class="CmbBox (strict)"() -> (reference out=w1083:refnum<vi>, "Value"=w1084:T2)  [unwired: 2 in, 1 out]
                    n527 = property on="Property Node" class="CmbBox (strict)"(reference=w1083, "Val(Sgnl)"=w1084) -> ()  [unwired: 1 in, 2 out]
                  }
                  frame Enabled {
                  }
                }
              }
            }
            n528 = case shown="0, Default" w1059 {
              tunnel: w1069 -> [w1075 _]
              frame 0, Default {
                # "Update MCListBox"
                n529 = property on="Current Record" class="DigNum (strict)"("Val(Sgnl)"=w1075) -> ()  [unwired: 2 in, 2 out]
              }
              frame 4 {
                # "Event already FIRED in Select Table"
              }
            }
            n530 = local write "Changed"(FALSE ("Changed")) -> ()
          }
          frame Enabled {
          }
        }
      }
    }
    "Statemachine" <- w85
  }
  n531 = disable-structure shown="Disabled" {
    frame Disabled {
      w1086 = "%Y-%m-%d %H:%M:%S"  # SQL Server datetime
      n532 = Get Date/Time In Seconds() -> (seconds since 1Jan1904=w1087:timestamp)
      n533 = Format Date/Time String(time format string (%c)=w1086, seconds (now)=w1087) -> (date/time string=w1085:string)  [unwired: 1 in]
      "datetime string" <- w1085
      n534 = Concatenate Strings("INSERT INTO " ("string"), "(TStamp)" ("string"), " values " ("string"), "('" ("string"), w1085, "')" ("string")) -> ()  [unwired: 1 in, 1 out]
    }
    frame Enabled {
    }
  }
  n535 = flat-sequence "Save Flags" {
    frame #0 {
      w1093 = FALSE
      # "Reset all Save Flags"
      n536 = local write "All Mandatory Fields Filled"(w1093) -> ()
      n537 = local write "Email Valid"(w1093) -> ()
      n538 = local write "Password Count Valid"(w1093) -> ()
      n539 = local write "Password Matched"(w1093) -> ()
    }
  }
  n540 = call <vilib>:"DB Tools Close Connection.vi"("error in (no error)"=w6, "connection reference"=w7) -> ("error out"=→"Close":errorcluster)  [unwired: 5 in]
